vi "Multi_Run_Prog.vi"(0 "Command filename":path, 1 "Setup mode":T9(ring)) -> ()   [LabVIEW 2013]
uses:
  Anemometry Sub Vis/Gen Trav/Traverse_cluster.ctl
  Anemometry Sub Vis/Gen Trav/Spacing.ctl
  Anemometry Sub Vis/Controls/Multi_run_mode.ctl
  Anemometry Sub Vis/Gen Trav/Route mapping/Route_Display_Mode.ctl
  Anemometry Sub Vis/Controls/User_Specific_mode.ctl
  Anemometry Sub Vis/Controls/Multi_Run_Case.ctl
  Anemometry Sub Vis/Gen Trav/Multi_Run_Status.ctl
  Anemometry Sub Vis/Controls/Tunnel_Coordinates.ctl
  Anemometry Sub Vis/Controls/Post_Process.ctl
  ADAM Client/Sub VIs/ADAM Controls/Traverse_Level_State.ctl
  ADAM Client/Sub VIs/ADAM Controls/Tunnel_speed_mode.ctl
  Anemometry Sub Vis/Controls/Overhead.ctl
  ADAM Client/Sub VIs/ADAM Controls/Remember_value_mode.ctl
  Anemometry Sub Vis/Gen Trav/Trav_mode.ctl
  ADAM Client/Sub VIs/ADAM Controls/Client_Source_Status.ctl
  ADAM Client/Sub VIs/ADAM Controls/Update_scan_value.ctl
  Anemometry Sub Vis/File/Setup_Filetype.ctl
  Anemometry Sub Vis/Globals/Meas_global.vi
  Anemometry Sub Vis/Globals/Trav_pos_global.vi
  Anemometry Sub Vis/Globals/Preference_global.vi
  Anemometry Sub Vis/Gen Trav/Route mapping/Route_mapping_global.vi
  ADAM Serial/Instrument drivers/Traverses/~subVIs/DriveConfigGlobal.vi
  Anemometry Sub Vis/Globals/Extra_Commands_Global.vi
panel:
  out "Last Row Run":i32
  in  "Stop after Repeats":bool
  in  "Jump Bad Positions":bool
  in  "Work in Tunnel Coordinates?":T1
  out "Current Overhead Factor":dbl format="%.3f"
  out "Estimated Completion time":string
  out "Max Tunnel Speed":dbl format="%.2f"
  out "Pause message":string
  in  "Pause":bool
  out "Non Starter":bool
  out "No of Rows":i32
  out "Status":T2
  in  "Synchronization Start No":i32=1 min=1 max=100
  out "Multi Run Case":T3
  out "Simulate/Run":T4
  in  "Display Mode":T5=enum."Display View on Crash"
  in  "stop":bool
  out "Currently on Row":i32
  in  "Table":T6[](array[typedef]) {"Row Duration (mins)" format="%#.1f"; "Row No" min=0; "Trace Gas Concentration (%)" min=0.0 format="%#.2f"; "Emission Rate (l/min)" format="%#.2f"; "Tunnel Speed" format="%#.2f"; "Start X" format="%#.2f"; "Start Y" format="%#.2f"; "Start Z" format="%#.2f"; "End X" format="%#.2f"; "End Y" format="%#.2f"; "End Z" format="%#.2f"; "Averaging time (min)" min=0.0 format="%#.2f"}
  # "X           Y            Z"
  # "Start"
  # "End"
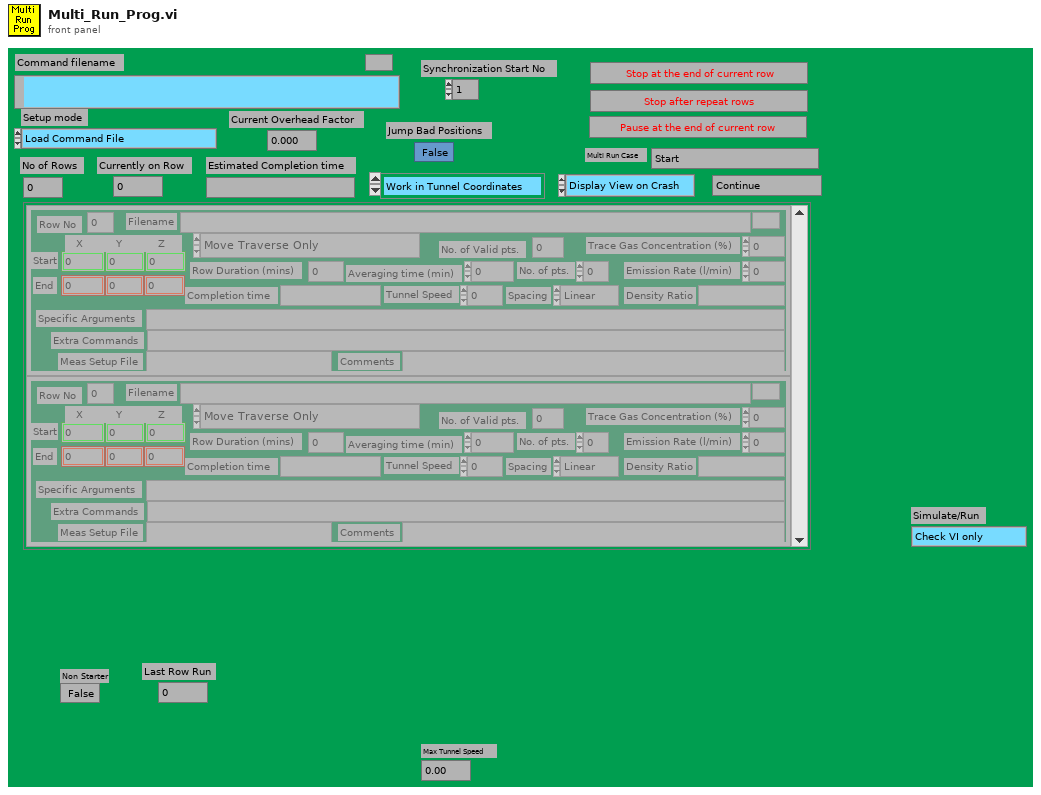
[diagram p1: front panel]
types:
  T1 = typedef "Tunnel_Coordinates.ctl" = enum16{"Work in Tunnel Coordinates", "Work in Model Coordinates"}
  T2 = typedef "Multi_Run_Status.ctl" = enum16{"Continue", "Jump to Next Point", "Jump to Next Row", "Jump To Fall Back", "Terminate Run"}
  T3 = typedef "Multi_Run_Case.ctl" = enum16{"Start", "Load Setup From File", "Has file been edited in Excel?", "Check Max Tunnel Speed", "Pre Check Row", "Check Rows", "Remove blank end rows", "Do results files already exist?", "FFID Bkgnd Measurements?", "First Save Setup file", "Setup Route checking", "Initialise Measurement Prog", "Input Current Position", "Experimental setup control", "Check source flowrates", "Setup for running mode", "Skip Blank Rows", "Which row to execute next", "Evaluate IF Statement", "Perform Measurement Setup", "Set Measurement Conditions", "Execute Row", "Calculate Row TIme", "Update time estimate", "Pause Multi Run Program", "Do Another Row?", "Find Next Fall Back Row", "Shut down source etc", "Email results to users", "Save run efficiency", "Remove Skipped Commands", "Show jumped positions", "Save Setup to File", "End"}
  T4 = typedef "User_Specific_mode.ctl" = enum16{"Check VI only", "Run VI"}
  T5 = typedef "Route_Display_Mode.ctl" = enum16{"Display View Always", "Display View on Crash"}
  T6 = typedef "Traverse_cluster.ctl" = cluster{"Start X":dbl, "Start Y":dbl, "Start Z":dbl, "End X":dbl, "End Y":dbl, "End Z":dbl, "No. of pts.":i32, "Spacing":T7, "Filename":path, "Tunnel Speed":dbl, "Averaging time (min)":dbl, "Extra Commands":string, "Specific Arguments":string, "Emission Rate (l/min)":dbl, "Trace Gas Concentration (%)":dbl, "Density Ratio":string, "Comments":string, "Row No":i32, "Row Type Selector":T8, "Completion time":string, "Row Duration (mins)":dbl, "No. of Valid pts.":i32, "Meas Setup File":string}
  T7 = typedef "Spacing.ctl" = enum16{"Linear", "Log", "Gauss", "Specified", "N/A"}
  T8 = typedef "Multi_run_mode.ctl" = enum16{"Move Traverse Only", "Set Tunnel Speed Only", "Set Source Only", "Set Measurement Conditions", "Single Measurement", "Vertical Profile", "Lateral Profile", "Longitudinal Profile", "Explore Volume", "Multi-Axis Profile", "Auto Calibrate", "Meas Fast FID Bkgnd", "Check Beam Power", "Scanning Valve Measurement", "Run VI Named:", "Set ADAM Ch", "Wait (minutes)", "Send Message", "Synchronize With:", "Fall Back to this Row", "Turn Off Row Repeating", "Blank Row", "Traverse 3D Volume"}
  T9 = enum16{"Load Command File", "Save Command File", "Check Multi Run Prog", "Check Multi Run Prog With Live Moves", "Run Multi Run Prog"}
  T10 = typedef "Post_Process.ctl" = enum16{"Take New Data", "Post Process Raw Data File"}
  T11 = typedef "Traverse_Level_State.ctl" = enum16{"Running", "Complete"}
  T12 = enum32{"existing file", "new file", "new or existing file", "existing dir", "new dir", "new or existing dir", "existing file (use LLBs)", "new file (use LLBs)", "new or existing file (use LLBs)", "new or existing file or directory (use LLBs)"}
  T13 = typedef "Tunnel_speed_mode.ctl" = enum16{"Set Speed", "Set Speed then wait", "Is tunnel speed allowable?"}
  T14 = enum16{"All Channel Names", "Valid Channel Names"}
  T15 = typedef "Overhead.ctl" = enum16{"Update total times", "Read Current Overhead", "Re Scale totals to 3 hrs", "Initialise totals to 3hr"}
  T16 = typedef "Remember_value_mode.ctl" = enum16{"Read only", "Read and Write"}
  T17 = typedef "Trav_mode.ctl" = enum16{"Move traverse", "Read traverse position", "Teach Position"}
  T18 = typedef "Client_Source_Status.ctl" = enum16{"Not Using", "Using", "Must Have"}
  T19 = typedef "Update_scan_value.ctl" = cluster{"Channel Name":string, "New Value":dbl}
  T20 = typedef "Setup_Filetype.ctl" = enum16{"Measurement Setups", "Calibration Setups", "General", "Results File Plotter Setups", "Speed Calib Tweaks"}
  T21 = typedef "AxisConfigCluster.ctl" = cluster{"Channel Properties":T22, "Static Drive Configuration":T23}
  T22 = typedef "DriveProperties.ctl" = cluster{"Channel Name":string, "Vel. Default":dbl, "Acc. Default":dbl, "Vel. Max":dbl, "Vel. Min":dbl, "Acc. Max":dbl, "Acc. Min":dbl, "Pulses/unit":dbl, "Address":u8, "Pulse Offset":i32, "Pos Tolerance":dbl, "Pulses/rev":dbl, "Backlash/Eng units":dbl, "Current Pos":dbl, "Ch Status":enum16{"Active", "Offline", "Simulate"}, "Port Name":string, "Axis Transform mode":string, "Metadata Ch Name":string, "Type":string}
  T23 = typedef "DriveStaticConfig.ctl" = cluster{"Correction Gain % (CG)":u16, "Dead Band (DB)":i32, "Dead Band Window (DW)":i32, "Encoder Resolution (ER)":i32, "Step Mode  (FSB)":u16, "Position Maintenance (FSC)":u16, "Stop on Stall (FSD)":u16, "Activate OP1 on stall (FSE)":u16, "Stop on Trigger 3 (FSF)":u16, "OP2 in Deadband (FSG)":u16, "Stall Detect (FSH)":u16, "Limit Disable (LD)":u16, "Motor Resolution (MR)":enum16{"200", "400", "1000", "2000", "4000", "5000", "10000", "12800", "18000", "20000", "21600", "25000", "25400", "25600", "36000", "50000", "278528", "425984", "507904", "614400", "655360", "819200", "1024000"}, "Limit Switch Sense (OSA)":u16, "Home Position (OSB)":u16, "Home Switch Sense (OSC)":u16, "Encoder Z for Home (OSD)":u16, "Reference edge of Home (OSH)":u16, "RS232 Echo Control (SSA)":u16, "Buffer at Limit (SSG)":u16, "Buffer at Stop (SSH)":u16, "Indexer Mode  (FSA)":u16, "Type":string, "ConfigString":string, "De Power Motor":enum16{"TRUE", "FALSE"}}
  T24 = typedef "Status_Cluster.ctl" = cluster{"Status":T2, "Error Type":string, "Error Description":string}
  T25 = typedef "Server_Comms.ctl" = enum16{"Server Link Healthy", "Do Not Link To Server"}
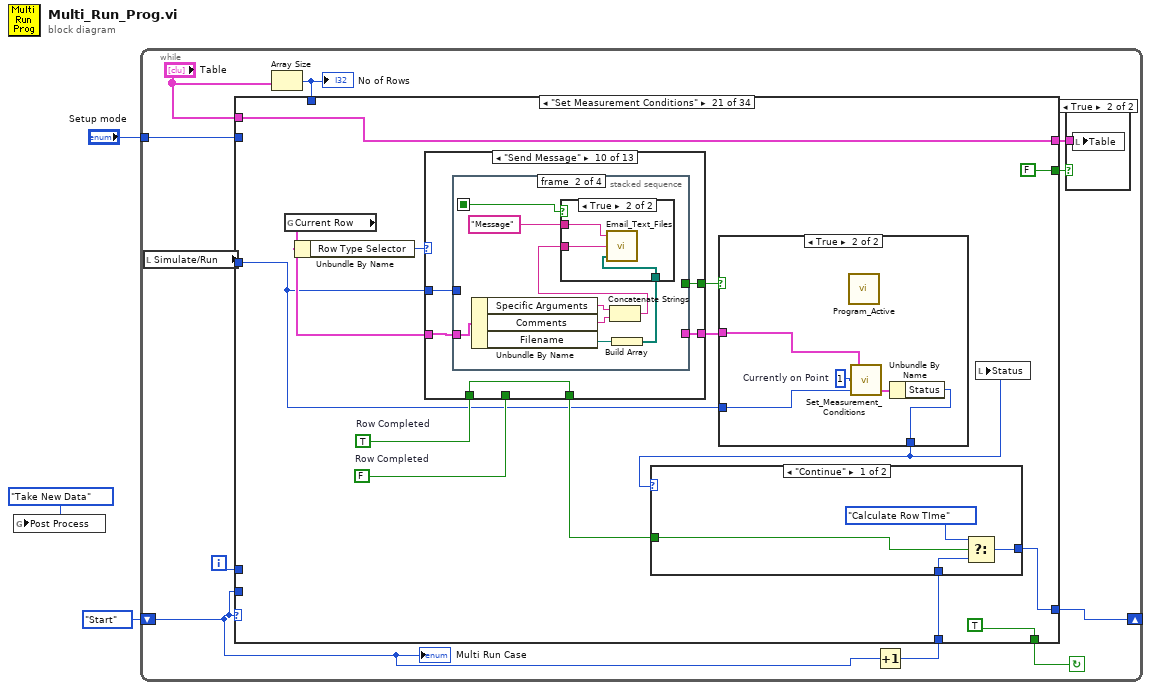
[diagram p0: block diagram]
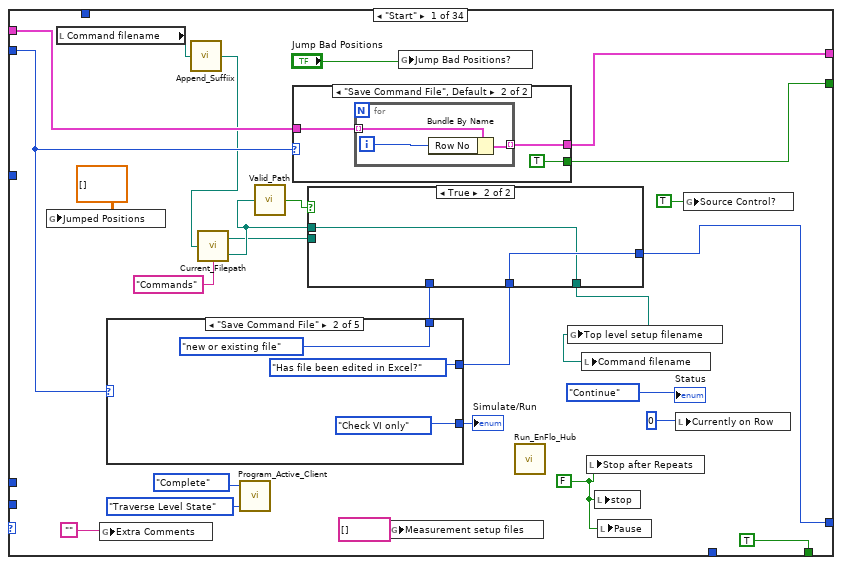
[diagram p3: hidden frame]
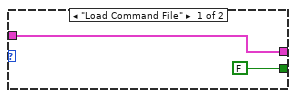
[diagram p4: hidden frame]
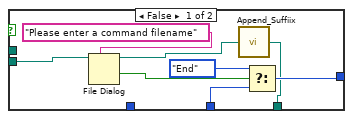
[diagram p5: hidden frame]
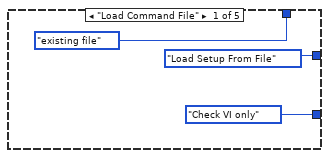
[diagram p6: hidden frame]
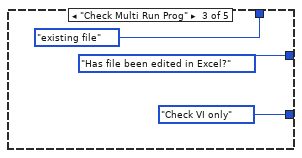
[diagram p7: hidden frame]
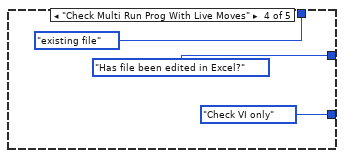
[diagram p8: hidden frame]
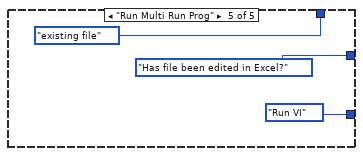
[diagram p9: hidden frame]
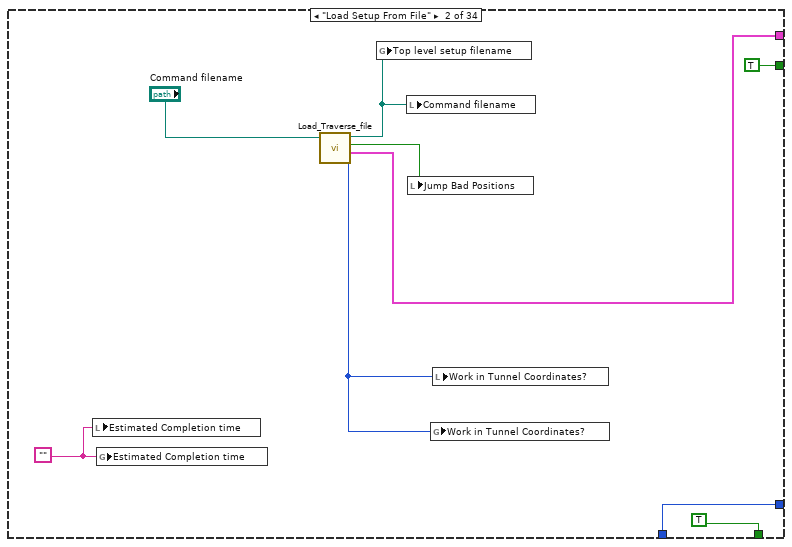
[diagram p10: hidden frame]
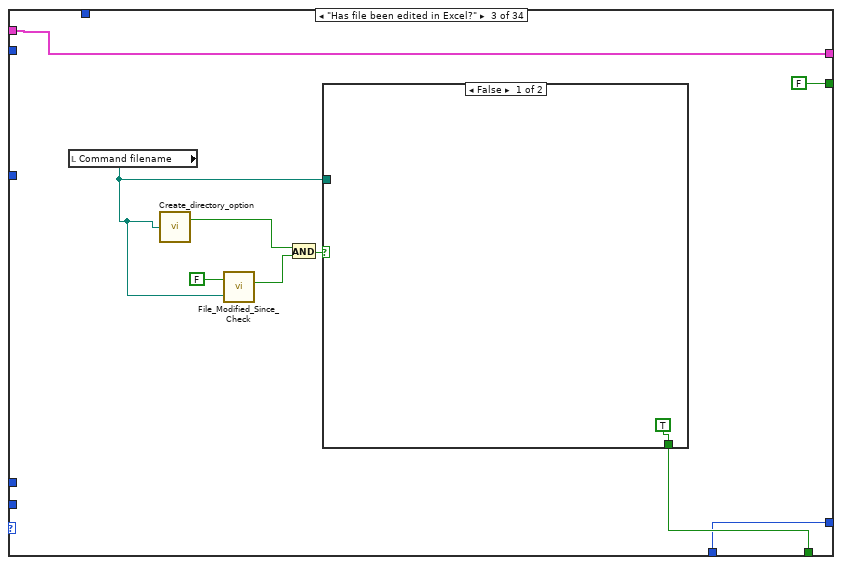
[diagram p11: hidden frame]
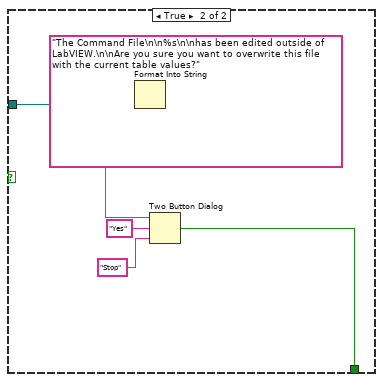
[diagram p12: hidden frame]
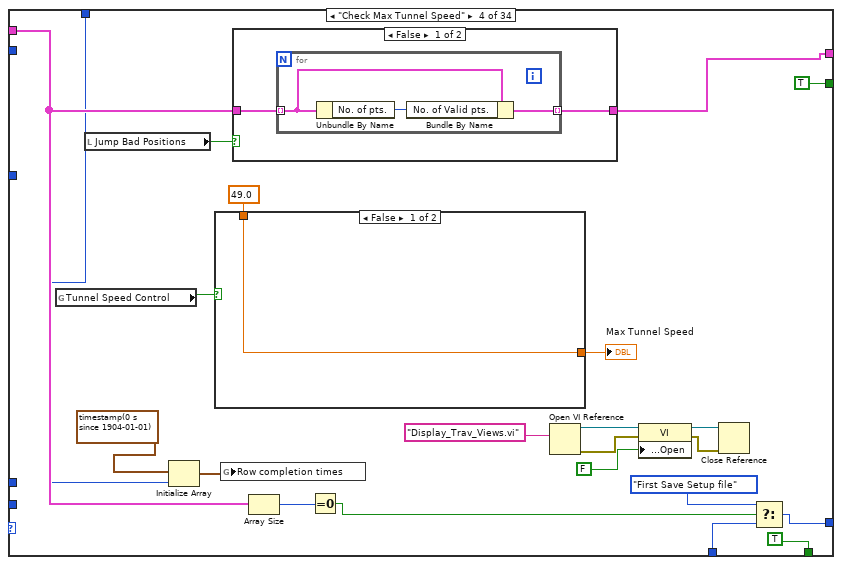
[diagram p13: hidden frame]
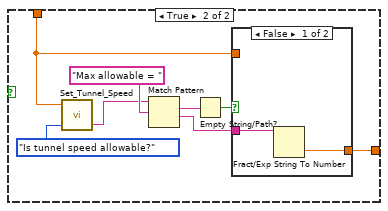
[diagram p15: hidden frame]
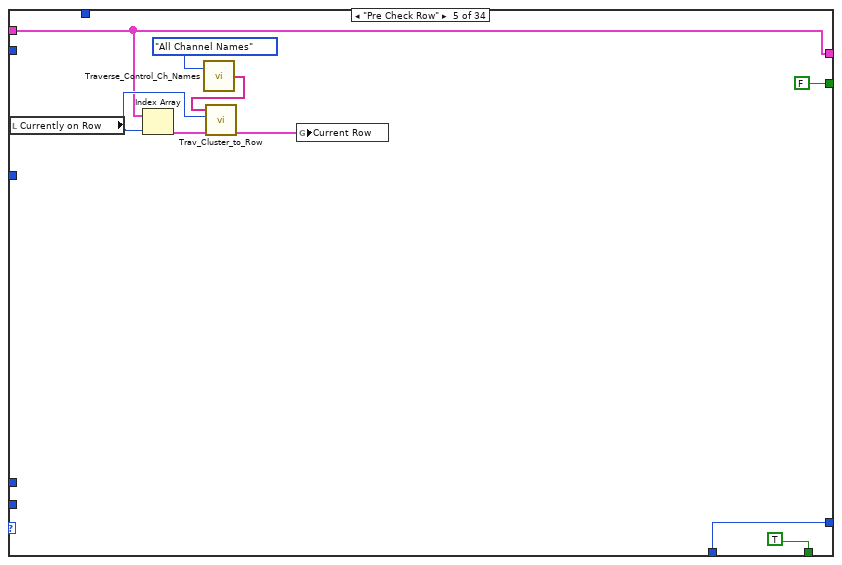
[diagram p17: hidden frame]
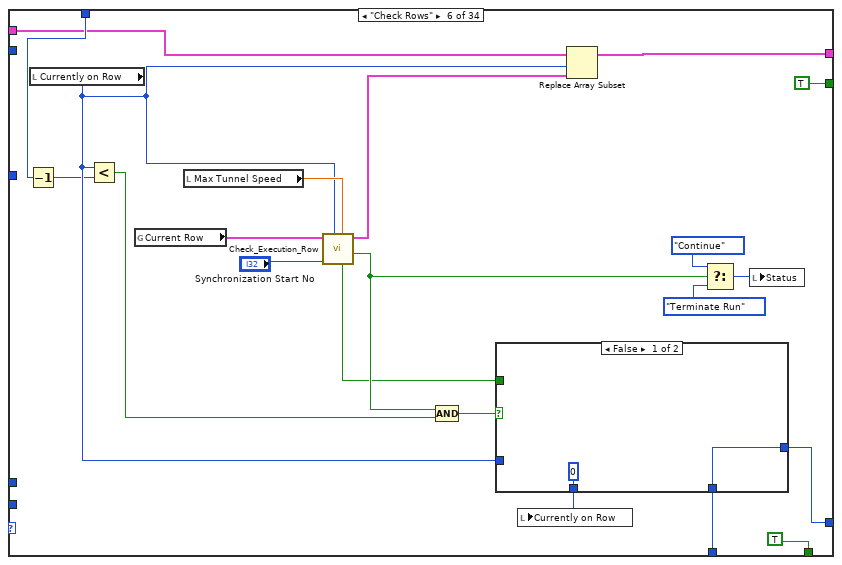
[diagram p18: hidden frame]
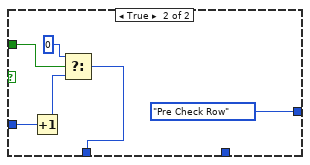
[diagram p19: hidden frame]
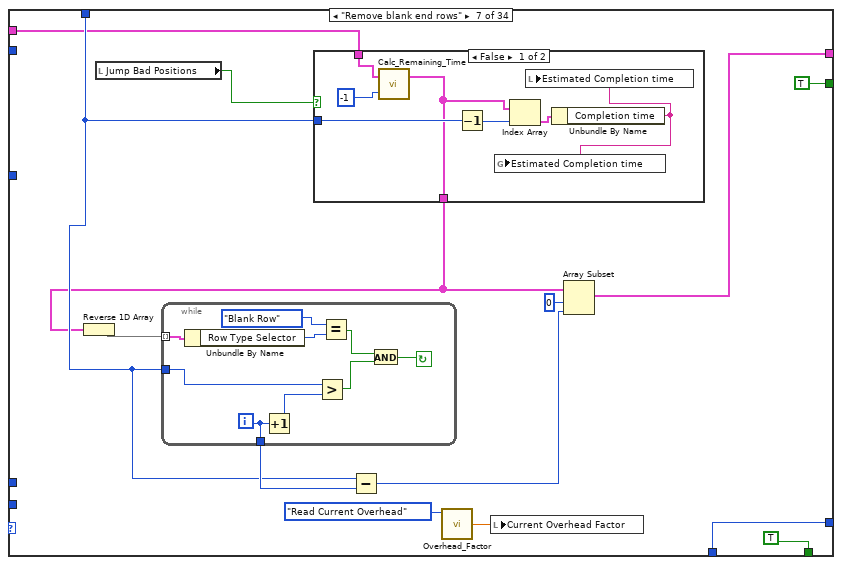
[diagram p20: hidden frame]
diagram:
  n1 = global write "Meas_global.vi" "Post Process"(Post_Process."Take New Data" ("Post Process")) -> ()
  n2 = while {
    shift-left: Multi_Run_Case."Start" ("Multi Run Case") -> [w10]
    shift-right: [w6] -> _
    tunnel: "Setup mode" -> [w13]
    i -> [w11]
    stop <- w14 continue-if-true
    n3 = local read "Simulate/Run"() -> (w7:T4)
    n4 = Array Size(array="Table") -> (size(s)=w5:i32)
    "No of Rows" <- w5
    n5 = Increment(x=w10) -> (x+1=w12:T3)
    n6 = case shown="\"Set Measurement Conditions\"" w10 {
      tunnel: [TRUE TRUE w87 TRUE TRUE TRUE TRUE TRUE TRUE TRUE TRUE ("Continue?") TRUE ("Continue?") TRUE TRUE TRUE w506 TRUE ("Continue?") TRUE ("Continue?") TRUE TRUE ("Continue?") TRUE TRUE TRUE TRUE TRUE TRUE TRUE TRUE TRUE TRUE TRUE TRUE TRUE FALSE] -> w14
      tunnel: w13 -> [w26 _ _ _ _ _ _ _ _ w395 _ _ _ _ _ _ _ _ _ _ _ _ _ _ _ _ _ _ _ _ _ _ w1254 _]
      tunnel: "Table" -> [w39 _ w84 w114 w142 w154 w179 w210 w368 w397 w419 w472 w477 w483 w493 w509 w580 w624 w740 w791 w803 w896 w932 w964 w1007 w1053 w1101 w1131 w1152 w1199 w1204 w1213 w1275 w1339]
      tunnel: w7 -> [_ _ _ _ _ _ _ w209 _ _ _ _ _ w487 w492 w508 _ w622 w737 w788 w801 w895 w930 w961 _ w1062 _ w1122 _ _ _ _ w1265 _]
      tunnel: w10 -> [_ _ _ _ _ _ _ _ _ _ _ _ _ _ _ _ _ _ _ _ _ _ _ _ _ _ _ _ _ _ _ _ _ _]
      tunnel: w12 -> [_ w80 w86 w112 w146 w156 w190 w214 w363 w394 w423 w470 w478 w482 w498 w511 w582 w620 w745 w792 w810 w893 w922 w966 w1010 _ _ w1115 w1154 w1201 w1207 w1221 w1273 w1338]
      tunnel: w11 -> [_ _ _ _ _ _ _ _ _ _ _ _ _ _ _ _ _ _ _ _ _ _ _ _ w1008 _ _ _ _ _ _ _ _ _]
      tunnel: [w37 w80 w86 w111 w146 w155 w190 w214 w363 w390 w423 w469 w478 w482 w495 w511 w582 w621 w744 w792 w811 w893 w922 w966 w1011 w1045 w1098 w1126 w1154 w1201 w1207 w1221 w1273 w1338] -> w6
      tunnel: [w25 TRUE FALSE ("Rows Added ?") TRUE ("Rows Added ?") FALSE TRUE TRUE FALSE FALSE TRUE FALSE FALSE FALSE FALSE FALSE TRUE FALSE ("Rows Added ?") FALSE ("Rows Added ?") FALSE FALSE ("Rows Added ?") FALSE FALSE FALSE TRUE ("Rows Added ?") FALSE FALSE FALSE FALSE FALSE FALSE TRUE TRUE TRUE FALSE] -> w8
      tunnel: w5 -> [_ _ _ w106 _ w160 w181 _ _ _ _ _ _ _ _ _ w583 w623 _ _ _ _ _ w960 _ w1048 _ _ _ _ _ _ _ _]
      tunnel: [w38 w81 w84 w116 w142 w163 w185 w210 w368 w398 w419 w472 w477 w483 w493 w507 w580 w625 w740 w791 w803 w896 w932 w963 w1007 w1053 w1101 w1131 w1152 w1199 w1203 w1213 w1274 w1339] -> w4
      frame "Start" {
        w23 = FALSE ("Measurment setup Found?")
        n7 = global write "Trav_pos_global.vi" "Jumped Positions"(dbl[][] [] ("Jumped Positions")) -> ()
        n8 = local read "Command filename"() -> (w29:path)
        n9 = global write "Meas_global.vi" "Extra Comments"("") -> ()
        n10 = case shown="\"Save Command File\"" w26 {
          tunnel: [User_Specific_mode."Check VI only" ("Simulate/Run") User_Specific_mode."Check VI only" ("Simulate/Run") User_Specific_mode."Check VI only" ("Simulate/Run") User_Specific_mode."Check VI only" ("Simulate/Run") User_Specific_mode."Run VI" ("Simulate/Run")] -> w40
          tunnel: [Multi_Run_Case."Load Setup From File" ("Multi Run Case") Multi_Run_Case."Has file been edited in Excel?" ("Multi Run Case") Multi_Run_Case."Has file been edited in Excel?" ("Multi Run Case") Multi_Run_Case."Has file been edited in Excel?" ("Multi Run Case") Multi_Run_Case."Has file been edited in Excel?" ("Multi Run Case")] -> w36
          tunnel: [T12."existing file" ("select mode (2)") T12."new or existing file" ("select mode (2)") T12."existing file" ("select mode (2)") T12."existing file" ("select mode (2)") T12."existing file" ("select mode (2)")] -> w24
          frame "Load Command File" {
          }
          frame "Save Command File" {
          }
          frame "Check Multi Run Prog" {
          }
          frame "Check Multi Run Prog With Live Moves" {
          }
          frame "Run Multi Run Prog" {
          }
        }
        "Simulate/Run" <- w40
        n11 = call "Append_Suffiix.vi"("Results file"=w29) -> ("appended path"=w18:path)
        n12 = call "Current_Filepath.vi"("Filename in"=w18, "Data Type"="Commands") -> ("Filename Out"=w17:path, "Directory"=w16:path)
        n13 = call "Program_Active_Client.vi"("Mode"=enum16{"Program Active", "Traverse Level State"}."Traverse Level State", "Traverse level State"=Traverse_Level_State."Complete") -> ()  [unwired: 1 in, 3 out]
        n14 = call "Valid_Path.vi"("Filename"=w17) -> ("Valid Path?"=w27:bool)
        n15 = case shown="\"Save Command File\", Default" w26 {
          tunnel: w39 -> [w43 w46]
          tunnel: [w43 w45] -> w38
          tunnel: [FALSE TRUE] -> w25
          frame "Load Command File" {
          }
          frame "Save Command File", Default {
            n16 = for {
              tunnel: w46 -> [w49] mode=indexing
              tunnel: [w48] -> w45 mode=indexing
              i -> [w47]
              n17 = Bundle By Name(cluster=w49, "Row No"=w47) -> (w48:T6)
            }
          }
        }
        n18 = case shown="True" w27 {
          tunnel: [w55 w59] -> w37
          tunnel: w36 -> [w56 w59]
          tunnel: w17 -> [_ w58]
          tunnel: [w54 w58] -> w28
          tunnel: w24 -> [_ _]
          tunnel: w16 -> [w50 _]
          frame False {
            n19 = File Dialog(7:"Please enter a command filename" ("prompt"), 11:w50) -> (1:w52:bool, 3:w53:path)  [unwired: 1 in, 6 out]
            n20 = call "Append_Suffiix.vi"("Results file"=w53) -> ("appended path"=w54:path)
            n21 = Select(t=Multi_Run_Case."End" ("Multi Run Case"), s=w52, f=w56) -> (s? t:f=w55:T3)
          }
          frame True {
          }
        }
        n22 = global write "Trav_pos_global.vi" "Measurement setup files"(string[] [] ("Measurement setup files")) -> ()
        n23 = global write "Trav_pos_global.vi" "Jump Bad Positions?"("Jump Bad Positions") -> ()
        n24 = call "Run_EnFlo_Hub.vi"() -> ()  [unwired: 8 out]
        n25 = global write "Trav_pos_global.vi" "Top level setup filename"(w28) -> ()
        n26 = local write "Command filename"(w28) -> ()
        n27 = local write "Stop after Repeats"(w23) -> ()
        n28 = local write "stop"(w23) -> ()
        n29 = local write "Pause"(w23) -> ()
        n30 = local write "Currently on Row"(0 ("Currently on Row")) -> ()
        n31 = global write "Trav_pos_global.vi" "Source Control?"(TRUE ("Source Control?")) -> ()
        "Status" <- Multi_Run_Status."Continue" ("Status")
      }
      frame "Load Setup From File" {
        w76 = ""
        n32 = local write "Estimated Completion time"(w76) -> ()
        n33 = global write "Trav_pos_global.vi" "Estimated Completion time"(w76) -> ()
        n34 = call "Load_Traverse_file.vi"("Setup filename"="Command filename") -> ("Setup filename Out"=w78:path, "Jump Bad Positions"=w75:bool, "Table"=w81:T6[], "Work in Tunnel Coordinates?"=w77:T1)  [unwired: 2 out]
        n35 = global write "Trav_pos_global.vi" "Top level setup filename"(w78) -> ()
        n36 = local write "Command filename"(w78) -> ()
        n37 = local write "Jump Bad Positions"(w75) -> ()
        n38 = global write "Trav_pos_global.vi" "Work in Tunnel Coordinates?"(w77) -> ()
        n39 = local write "Work in Tunnel Coordinates?"(w77) -> ()
      }
      frame "Has file been edited in Excel?" {
        n40 = local read "Command filename"() -> (w88:path)
        n41 = call "Create_directory_option.vi"("Filename"=w88) -> ("Path is to existing File"=w91:bool)  [unwired: 1 out]
        n42 = call "File_Modified_Since_Check.vi"("Pathname"=w88, "Just Modified?"=FALSE) -> ("Modified?"=w90:bool)
        n43 = And(x=w91, y=w90) -> (x .and. y?=w92:bool)
        n44 = case shown="False" w92 {
          tunnel: w88 -> [_ w99]
          tunnel: [TRUE ("T button?") w94] -> w87
          frame False {
          }
          frame True {
            n45 = Format Into String(format string="The Command File\n\n%s\n\nhas been edited outside of LabVIEW.\n\nAre you sure you want to overwrite this file  with the current table values?" ("Format String"), w99) -> (resulting string=w97:string)  [unwired: 2 in, 1 out]
            n46 = Two Button Dialog(message=w97, 1:"Stop" ("F button name (\"Cancel\")"), 2:"Yes" ("T button name (\"OK\")")) -> (T button?=w94:bool)
          }
        }
      }
      frame "Check Max Tunnel Speed" {
        n47 = global read "Preference_global.vi" "Tunnel Speed Control"() -> (w117:bool)
        n48 = local read "Jump Bad Positions"() -> (w115:bool)
        n49 = Initialize Array(timestamp(0 s since 1904-01-01) ("seconds since 1Jan1904"), w106) -> (w107:timestamp[])
        n50 = case shown="False" w117 {
          tunnel: 49.0 ("Tunnel Velocity m/s") -> [w128 w129]
          tunnel: [w128 w131] -> w119
          frame False {
          }
          frame True {
            n51 = call "Set_Tunnel_Speed.vi"("Mode"=Tunnel_speed_mode."Is tunnel speed allowable?", "Tunnel Velocity m/s"=w129) -> ("Error String"=w134:string)  [unwired: 1 in, 2 out]
            n52 = Match Pattern(string=w134, regular expression="Max allowable = ") -> (match substring=w133:string, after substring=w130:string)  [unwired: 3 out]
            n53 = Empty String/Path?(string/path=w133) -> (empty?=w132:bool)
            n54 = case shown="False" w132 {
              tunnel: [w137 w139] -> w131
              tunnel: w129 -> [_ w139]
              tunnel: w130 -> [w138 _]
              frame False {
                n55 = Fract/Exp String To Number(string=w138) -> (number=w137:dbl)  [unwired: 4 out]
              }
              frame True {
              }
            }
          }
        }
        "Max Tunnel Speed" <- w119
        n56 = global write "Trav_pos_global.vi" "Row completion times"(w107) -> ()
        n57 = case shown="False" w115 {
          tunnel: w114 -> [w123 w127]
          tunnel: [w122 w127] -> w116
          frame False {
            n58 = for {
              tunnel: w123 -> [w125] mode=indexing
              tunnel: [w124] -> w122 mode=indexing
              n59 = Unbundle By Name(w125) -> ("No. of pts."=w126:i32)
              n60 = Bundle By Name(cluster=w125, "No. of Valid pts."=w126) -> (w124:T6)
            }
          }
          frame True {
          }
        }
        n61 = Array Size(array=w114) -> (size(s)=w113:i32)
        n62 = Equal To 0?(x=w113) -> (x = 0?=w110:bool)
        n63 = Open VI Reference(vi path="Display_Trav_Views.vi" ("VI path")) -> (vi reference=w105:refnum<vi>, error out=w104:errorcluster)  [unwired: 1 in, 4 out]
        n64 = property class="VI"(reference=w105, error in=w104, "Front Panel Window:Open"=FALSE) -> (reference out=w102:refnum<vi>, error out=w101:errorcluster)
        n65 = Close Reference(reference=w102, error in (no error)=w101) -> ()  [unwired: 1 out]
        n66 = Select(t=Multi_Run_Case."First Save Setup file" ("Multi Run Case"), s=w110, f=w112) -> (s? t:f=w111:T3)
      }
      frame "Pre Check Row" {
        n67 = local read "Currently on Row"() -> (w143:i32)
        n68 = Index Array(array=w142, index=w143) -> (element=w144:T6)
        n69 = call "Traverse_Control_Ch_Names.vi"("Mode"=T14."All Channel Names") -> ("Channel names"=w140:string[])  [unwired: 1 in]
        n70 = call "Trav_Cluster_to_Row.vi"("Traverse line in"=w144, "Row Number"=w143, "Channel names"=w140) -> ("Traverse line Out"=w145:T6)  [unwired: 4 out]
        n71 = global write "Trav_pos_global.vi" "Current Row"(w145) -> ()
      }
      frame "Check Rows" {
        n72 = Decrement(x=w160) -> (x-1=w151:i32)
        n73 = local read "Currently on Row"() -> (w152:i32)
        n74 = Less?(x=w152, y=w151) -> (x < y?=w159:bool)
        n75 = global read "Trav_pos_global.vi" "Current Row"() -> (w149:T6)
        n76 = local read "Max Tunnel Speed"() -> (w162:dbl)
        n77 = call "Check_Execution_Row.vi"("Execution Row"=w149, "Synchronization Start No"="Synchronization Start No", "Row Index"=w152, "Max Tunnel Speed"=w162) -> ("Editted Row"=w150:bool, "Execution Row Out"=w153:T6, "Continue?"=w161:bool)  [unwired: 1 in, 3 out]
        n78 = Compound Arithmetic op=AND(w161, w159) -> (w158:bool)
        n79 = case shown="False" w158 {
          tunnel: [0 w173] -> w157
          tunnel: w152 -> [_ w177]
          tunnel: w156 -> [w171 _]
          tunnel: [w171 Multi_Run_Case."Pre Check Row" ("Multi Run Case")] -> w155
          tunnel: w150 -> [_ w175]
          frame False {
          }
          frame True {
            n80 = Increment(x=w177) -> (x+1=w174:i32)
            n81 = Select(t=0, s=w175, f=w174) -> (s? t:f=w173:i32)
          }
        }
        n82 = local write "Currently on Row"(w157) -> ()
        n83 = Replace Array Subset(array=w154, new element=w153, index=w152) -> (w163:T6[])
        n84 = Select(t=Multi_Run_Status."Continue" ("Status"), s=w161, f=Multi_Run_Status."Terminate Run" ("Status")) -> (s? t:f=w167:T2)
        n85 = local write "Status"(w167) -> ()
      }
      frame "Remove blank end rows" {
        n86 = local read "Jump Bad Positions"() -> (w178:bool)
        n87 = case shown="False" w178 {
          tunnel: w181 -> [w196 _]
          tunnel: w179 -> [w195 w199]
          tunnel: [w193 w199] -> w180
          frame False {
            n88 = call "Calc_Remaining_Time.vi"("Currently on Row"=-1 ("Start Index"), "Table In"=w195) -> ("Table Out"=w193:T6[])  [unwired: 1 out]
            n89 = Decrement(x=w196) -> (x-1=w198:i32)
            n90 = Index Array(array=w193, index=w198) -> (element=w197:T6)
            n91 = Unbundle By Name(w197) -> ("Completion time"=w192:string)
            n92 = global write "Trav_pos_global.vi" "Estimated Completion time"(w192) -> ()
            n93 = local write "Estimated Completion time"(w192) -> ()
          }
          frame True {
          }
        }
        n94 = Reverse 1D Array(array=w180) -> (reversed array=w189:T6[])
        n95 = while {
          tunnel: [w200] -> w187
          tunnel: w181 -> [w204]
          tunnel: w189 -> [w208] mode=indexing
          i -> [w200]
          stop <- w201 continue-if-true
          n96 = Unbundle By Name(w208) -> ("Row Type Selector"=w206:T8)
          n97 = Increment(x=w200) -> (x+1=w205:i32)
          n98 = Greater?(x=w204, y=w205) -> (0:w203:bool)
          n99 = Equal?(x=Multi_run_mode."Blank Row" ("Row Type Selector"), y=w206) -> (x = y?=w202:bool)
          n100 = And(x=w202, y=w203) -> (x .and. y?=w201:bool)
        }
        n101 = Subtract(x=w181, y=w187) -> (x-y=w186:i32)
        n102 = call "Overhead_Factor.vi"("Mode"=Overhead."Read Current Overhead") -> ("Current Overhead Factor"=w182:dbl)  [unwired: 3 in]
        n103 = local write "Current Overhead Factor"(w182) -> ()
        n104 = Array Subset(array=w180, index=0 ("Array Index"), length=w186) -> (w185:T6[])
      }
      frame "Do results files already exist?" {
        n105 = for {
          tunnel: w210 -> [w226] mode=indexing
          tunnel: [w224] -> w216 mode=indexing
          shift-right: [w220] -> _
          shift-left: path[] [] -> [w221]
          tunnel: w209 -> [w218]
          n106 = Unbundle By Name(w226) -> ("Specific Arguments"=w217:string, "Emission Rate (l/min)"=w225:dbl, "Row Type Selector"=w223:T8, "Filename"=w222:path)
          n107 = while {
            shift-left: w221 -> [w234]
            shift-right: [w233] -> w220
            tunnel: w222 -> [w235]
            tunnel: w223 -> [w239]
            shift-left: 0 -> [w240]
            shift-right: [w236] -> _
            tunnel: w218 -> [w230]
            shift-right: [w229] -> _
            shift-left: _ -> [w228]
            tunnel: w217 -> [w227]
            stop <- w238 continue-if-true
            n108 = Increment(x=w240) -> (x+1=w237:i32)
            n109 = case shown="0, Default" w240 {
              tunnel: w239 -> [w249 _ _ _ _ _ _ _ _ _ _ _]
              tunnel: [w244 w269 w274 w281 w286 TRUE ("exists?") TRUE ("exists?") FALSE ("exists?") FALSE ("exists?") TRUE ("true") w343 w356] -> w238
              tunnel: w237 -> [w251 w272 w277 w280 w287 w292 w303 w314 w325 w329 w341 _]
              tunnel: [w251 w272 w277 w280 w287 w290 w302 w314 w325 w330 w341 w355] -> w236
              tunnel: [w250 w271 w276 w279 w284 w300 w311 w316 w318 w327 w345 w361] -> w233
              tunnel: w234 -> [w250 w271 w276 w279 w285 w300 w311 w316 w318 w327 w345 w361]
              tunnel: w235 -> [w243 _ _ _ _ _ _ _ _ _ _ _]
              tunnel: 7 -> [_ _ _ _ _ _ _ _ _ w328 _ w355]
              tunnel: 9 -> [_ _ _ _ _ w291 _ _ _ _ _ _]
              tunnel: w230 -> [_ _ _ _ _ _ _ _ _ _ w344 _]
              tunnel: [w242 w268 w273 w278 w283 w288 w301 w312 w317 w326 w342 w354] -> w229
              tunnel: w228 -> [_ w268 w273 w278 w283 w288 w301 w312 w317 w326 w342 w354]
              tunnel: w227 -> [w241 _ _ _ _ _ _ _ _ _ _ _]
              frame 0, Default {
                n110 = case shown="\"Send Message\"" w249 {
                  tunnel: [TRUE w259 FALSE FALSE] -> w246
                  tunnel: w243 -> [w252 w258 w264 w266]
                  tunnel: w241 -> [_ w256 _ _]
                  tunnel: [w252 w258 w264 w266] -> w242
                  frame "Move Traverse Only", Default {
                  }
                  frame "Run VI Named:" {
                    n111 = Match Pattern(string=w256, regular expression=";") -> (before substring=w255:string)  [unwired: 4 out]
                    n112 = call <vilib>:"Trim Whitespace.vi"("string"=w255) -> ("trimmed string"=w254:string)  [unwired: 1 in]
                    n113 = Equal?(x=w254, y="Pressure_Tapped_Cube.vi") -> (x = y?=w260:bool)
                    n114 = Equal?(x=w254, y="Take_Data_on_the_Move.vi") -> (x = y?=w261:bool)
                    n115 = Or(x=w260, y=w261) -> (x .or. y?=w259:bool)
                  }
                  frame "Auto Calibrate" {
                  }
                  frame "Send Message" {
                  }
                }
                n116 = local read "Status"() -> (w247:T2)
                n117 = Not Equal?(x=Multi_Run_Status."Terminate Run" ("Status"), y=w247) -> (x != y?=w245:bool)
                n118 = And(x=w246, y=w245) -> (x .and. y?=w244:bool)
              }
              frame 1 {
                n119 = Not Equal?(x=path "", y=w268) -> (x != y?=w269:bool)
              }
              frame 2 {
                n120 = Not Equal?(x=w273, y=path "") -> (x != y?=w274:bool)
              }
              frame 3 {
                n121 = Search 1D Array(1D array=w279, element=w278) -> (index of element=w282:i32)  [unwired: 1 out]
                n122 = Less Than 0?(x=w282) -> (x < 0?=w281:bool)
              }
              frame 4 {
                n123 = Build Array (concatenate)(w285, w283) -> (w284:path[])
                n124 = call "Does_file_exist_(simple).vi"("Pathname"=w283) -> ("exists?"=w286:bool)
              }
              frame 5 {
                n125 = Path To String(path=w288) -> (string=w299:string)
                n126 = global read "Meas_global.vi" "Start Time of experiment"() -> (w294:dbl)
                n127 = Concatenate Strings(w299, "Append" ("Substring")) -> (w297:string)
                n128 = call "Remember_value.vi"("Mode"=Remember_value_mode."Read only", "Ch name"=w297) -> ("Output Value"=w295:dbl)  [unwired: 1 in]
                n129 = Not Equal?(x=w294, y=w295) -> (x != y?=w293:bool)
                n130 = Select(t=w292, s=w293, f=w291) -> (s? t:f=w290:i32)
              }
              frame 6 {
                n131 = Increment(x=w303) -> (x+1=w304:i32)
                n132 = Format Into String(format string="The results filename \"%s\" already exists.\nDo you wish to append to this file during the run?" ("Format String"), w301) -> (resulting string=w308:string)  [unwired: 2 in, 1 out]
                n133 = Two Button Dialog(message=w308, 1:"Abort Run" ("F button name (\"Cancel\")"), 2:"Append" ("T button name (\"OK\")")) -> (T button?=w305:bool)
                n134 = Select(t=w304, s=w305, f=w303) -> (s? t:f=w302:i32)
              }
              frame 7 {
                n135 = local write "Status"(Multi_Run_Status."Terminate Run" ("Status")) -> ()
              }
              frame 8 {
                n136 = Path To String(path=w317) -> (string=w324:string)
                n137 = Concatenate Strings(w324, "Append" ("Substring")) -> (w322:string)
                n138 = global read "Meas_global.vi" "Start Time of experiment"() -> (w319:dbl)
                n139 = call "Remember_value.vi"("Mode"=Remember_value_mode."Read and Write", "Input Value"=w319, "Ch name"=w322) -> ()  [unwired: 1 out]
              }
              frame 9 {
                n140 = call "Read_File_Simple.vi"("Filename"=w326) -> ("string"=w333:string)  [unwired: 2 in, 7 out]
                n141 = call "Is_it_a_Results_File.vi"("character string"=w333) -> ("Results File?"=w332:bool)  [unwired: 2 out]
                n142 = case shown="True" w332 {
                  tunnel: w326 -> [w336 _]
                  tunnel: [w334 w340] -> w330
                  tunnel: w329 -> [_ w340]
                  tunnel: w328 -> [w334 _]
                  frame False {
                    n143 = Path To String(path=w336) -> (string=w338:string)
                    n144 = Format Into String(format string="The File %s is not in the correct Results file format.\nCheck that it is tab delimited rather than excel format, or choose another file." ("Format String"), w338) -> (resulting string=w335:string)  [unwired: 2 in, 1 out]
                    n145 = One Button Dialog(message=w335, button name ("OK")="Stop") -> ()  [unwired: 1 out]
                  }
                  frame True {
                  }
                }
              }
              frame 10 {
                n146 = case shown="\"Check VI only\", Default" w344 {
                  tunnel: w342 -> [_ w353]
                  tunnel: [FALSE ("exists?") w347] -> w343
                  frame "Check VI only", Default {
                  }
                  frame "Run VI" {
                    n147 = call "Open_File_for_write.vi"("append to file? (new file:F)"=TRUE, "file path"=w353) -> ("error out"=w351:errorcluster, "refnum"=w352:refnum<file>)  [unwired: 1 in, 7 out]
                    n148 = Unbundle By Name(w351) -> ("code"=w350:i32)
                    n149 = Close File(refnum=w352, error in=w351) -> ()  [unwired: 2 out]
                    n150 = Equal?(x=10 ("code"), y=w350) -> (x = y?=w347:bool)
                  }
                }
              }
              frame 11 {
                n151 = Path To String(path=w354) -> (string=w359:string)
                n152 = Format Into String(format string="The File %s is already open in another application." ("Format String"), w359) -> (resulting string=w358:string)  [unwired: 2 in, 1 out]
                n153 = One Button Dialog(message=w358, button name ("OK")="Stop") -> (true=w356:bool)
              }
            }
          }
          n154 = Greater Than 0?(x=w225) -> (x > 0?=w224:bool)
        }
        n155 = Or Array Elements(Boolean array=w216) -> (logical OR=w212:bool)
        n156 = global write "Trav_pos_global.vi" "Source Control?"(w212) -> ()
      }
      frame "FFID Bkgnd Measurements?" {
        n157 = for {
          tunnel: w368 -> [w384] mode=indexing
          tunnel: [w372] -> w367 mode=indexing
          tunnel: [w373] -> w366 mode=indexing
          n158 = Unbundle By Name(w384) -> ("Row Type Selector"=w378:T8, "Specific Arguments"=w380:string)
          n159 = call "Get_array_values_fr_String.vi"("String Value"=w380) -> ("String array"=w381:string[])  [unwired: 1 out]
          n160 = Index Array(array=w381, index=0 ("Index")) -> (element=w377:string)
          n161 = Equal?(x=Multi_run_mode."Auto Calibrate" ("Row Type Selector"), y=w378) -> (x = y?=w374:bool)
          n162 = Equal?(x=w377, y="Concentration") -> (x = y?=w375:bool)
          n163 = Equal?(x=Multi_run_mode."Meas Fast FID Bkgnd" ("Row Type Selector"), y=w378) -> (x = y?=w372:bool)
          n164 = And(x=w374, y=w375) -> (x .and. y?=w373:bool)
        }
        n165 = Or Array Elements(Boolean array=w367) -> (logical OR=w364:bool)
        n166 = Or Array Elements(Boolean array=w366) -> (logical OR=w365:bool)
        n167 = Compound Arithmetic op=AND(invert w364, w365) -> (w362:bool)
        n168 = case shown="True" w362 {
          frame False {
          }
          frame True {
            n169 = One Button Dialog(message="This run automatically calibrates the Fast FID but does not have a Meas Fast FID Bkgnd row" ("format string")) -> ()  [unwired: 2 out]
          }
        }
      }
      frame "First Save Setup file" {
        w385 = -1 ("Currently on Row")
        n170 = case shown="\"Check Multi Run Prog\"" w395 {
          tunnel: [w402 w404 w406 Multi_Run_Case."End" ("Multi Run Case") Multi_Run_Case."End" ("Multi Run Case")] -> w389
          tunnel: w394 -> [w402 w404 w406 _ _]
          tunnel: [w403 w405 w407 w408 w410] -> w388
          frame "Run Multi Run Prog" {
            w403 = FALSE  # Live Traverse Preview?
          }
          frame "Check Multi Run Prog With Live Moves" {
            w405 = TRUE  # Live Traverse Preview?
          }
          frame "Check Multi Run Prog" {
            w407 = FALSE  # Live Traverse Preview?
          }
          frame "Load Command File" {
            w408 = FALSE  # Live Traverse Preview?
          }
          frame "Save Command File" {
            w410 = FALSE  # Live Traverse Preview?
          }
        }
        n171 = local read "Command filename"() -> (w396:path)
        n172 = global write "Trav_pos_global.vi" "Work in Tunnel Coordinates?"("Work in Tunnel Coordinates?") -> ()
        n173 = local write "Currently on Row"(w385) -> ()
        n174 = local write "Last Row Run"(w385) -> ()
        n175 = local read "Jump Bad Positions"() -> (w386:bool)
        n176 = call "Save_Trav_setup.vi"("Work in Tunnel Coordinates?"="Work in Tunnel Coordinates?", "Trav Table"=w397, "Jump Bad Positions"=w386, "Setup filename"=w396) -> ("Trav Table Out"=w398:T6[])  [unwired: 1 out]
        n177 = global write "Meas_global.vi" "Extra Comments"("") -> ()
        n178 = global write "Trav_pos_global.vi" "Live Traverse Preview?"(w388) -> ()
        n179 = local read "Status"() -> (w391:T2)
        n180 = case shown="\"Continue\"" w391 {
          tunnel: [w400 Multi_Run_Case."End" ("Multi Run Case")] -> w390
          tunnel: w389 -> [w400 _]
          frame "Continue" {
          }
          frame "Jump to Next Point", Default {
          }
        }
      }
      frame "Setup Route checking" {
        w415 = string[] []
        n181 = global read "Trav_pos_global.vi" "Work in Tunnel Coordinates?"() -> (w416:T1)
        n182 = for {
          tunnel: w419 -> [w459] mode=indexing
          shift-right: [w450] -> w417
          shift-left: string[] [] -> [w451]
          n183 = Unbundle By Name(w459) -> ("Extra Commands"=w452:string, "Start X"=w456:dbl, "Start Y"=w455:dbl, "Start Z"=w454:dbl)
          n184 = Build Array(w456, w455, w454) -> (w457:dbl[])
          n185 = Not A Number/Path/Refnum?(number/path/refnum=w457) -> (NaN/Path/Refnum?=w458:bool[])
          n186 = Or Array Elements(Boolean array=w458) -> (logical OR=w453:bool)
          n187 = case shown="False" w453 {
            tunnel: w452 -> [w463 _]
            tunnel: w451 -> [w462 w464]
            tunnel: [w461 w464] -> w450
            frame False {
              n188 = call "Which_Trav_Setup.vi"("Extra Command String"=w463) -> ("Traverse Setups"=w460:string[])
              n189 = Build Array (concatenate)(w462, w460) -> (w461:string[])
            }
            frame True {
            }
          }
        }
        n190 = call "Analyse_string_array.vi"("String array"=w417) -> ("Unique strings"=w412:string[])  [unwired: 2 out]
        n191 = for {
          tunnel: w412 -> [w429] mode=indexing
          tunnel: w416 -> [w428]
          shift-right: [w427] -> w413
          shift-left: w415 -> [w426]
          shift-right: [w424] -> w414
          shift-left: w415 -> [w425]
          n192 = stacked-sequence {
            tunnel: w429 -> [w433 w438]
            tunnel: w428 -> [w430 _]
            tunnel: [_ w437] -> w427
            tunnel: w426 -> [_ w436]
            tunnel: w425 -> [_ w435]
            tunnel: [_ w434] -> w424
            frame #0 {
              n193 = call "3D_Traverse_move.vi"("Mode"=Trav_mode."Read traverse position", "Work in Tunnel Coordinates"=w430, "Simulate/Run"=User_Specific_mode."Run VI", "Traverse name"=w433) -> ()  [unwired: 5 in, 7 out]
            }
            frame #1 {
              n194 = global read "DriveConfigGlobal.vi" "Configurations"() -> (w439:T21[])
              n195 = for {
                tunnel: w439 -> [w449] mode=indexing
                tunnel: w438 -> [w446]
                shift-right: [w444] -> w437
                shift-left: w436 -> [w445]
                shift-right: [w440] -> w434
                shift-left: w435 -> [w441]
                i -> [w448]
                n196 = Unbundle By Name(w449) -> ("Channel Properties.Metadata Ch Name"=w443:string)
                n197 = Format Into String(format string="%d", initial string=w446, w448) -> (resulting string=w442:string)  [unwired: 1 in, 1 out]
                n198 = Build Array (concatenate)(w445, w443) -> (w444:string[])
                n199 = Build Array (concatenate)(w441, w442) -> (w440:string[])
              }
            }
          }
        }
        n200 = global write "Trav_pos_global.vi" "ADAM Positions Ch names"(w413) -> ()
        n201 = global write "Route_mapping_global.vi" "Display Mode"("Display Mode") -> ()
        n202 = global write "Trav_pos_global.vi" "Route checking Chs"(w414) -> ()
        n203 = global write "Trav_pos_global.vi" "Traverses to Move"(w412) -> ()
      }
      frame "Initialise Measurement Prog" {
        n204 = for {
          tunnel: w472 -> [w476] mode=indexing
          tunnel: [w475] -> w466 mode=indexing
          n205 = Unbundle By Name(w476) -> ("Meas Setup File"=w475:string)
        }
        n206 = call "Analyse_string_array.vi"("String array"=w466) -> ("Unique strings"=w465:string[])  [unwired: 1 in, 1 out]
        n207 = call "Perform_Meas_Setup.vi"("Simulate/Run"=User_Specific_mode."Check VI only", "String array"=w465) -> ("Continue?"=w467:bool)  [unwired: 1 out]
        n208 = Select(t=w470, s=w467, f=Multi_Run_Case."End" ("Multi Run Case")) -> (s? t:f=w469:T3)
      }
      frame "Input Current Position" {
        n209 = call "Save_ADAM_Table_Locally.vi"() -> ()  [unwired: 12 in]
      }
      frame "Experimental setup control" {
        n210 = global read "Trav_pos_global.vi" "Source Control?"() -> (w484:bool)
        n211 = Equal?(x=w487, y=User_Specific_mode."Run VI" ("Simulate/Run")) -> (x = y?=w486:bool)
        n212 = Or(x=w484, y=w486) -> (x .or. y?=w485:bool)
        n213 = case shown="True" w485 {
          tunnel: w484 -> [_ w491]
          frame False {
          }
          frame True {
            n214 = call "Exp_Setup_Control_remote.vi"("Dispersion?"=w491) -> ()  [unwired: 3 out]
          }
        }
        n215 = global write "Trav_pos_global.vi" "FFID Background"(T6 {"Start X"=nan, "Start Y"=nan, "Start Z"=nan, "End X"=nan, "End Y"=nan, "End Z"=nan, "No. of pts."=0, "Spacing"=enum."Linear", "Filename"=path "", "Tunnel Speed"=nan, "Averaging time (min)"=nan, "Extra Commands"="", "Specific Arguments"="", "Emission Rate (l/min)"=nan, "Trace Gas Concentration (%)"=nan, "Density Ratio"="", "Comments"="", "Row No"=0, "Row Type Selector"=enum."Blank Row", "Completion time"="", "Row Duration (mins)"=nan, "No. of Valid pts."=0, "Meas Setup File"=""} ("FFID Background")) -> ()
      }
      frame "Check source flowrates" {
        n216 = case shown="\"Check VI only\", Default" w492 {
          tunnel: w493 -> [_ w502]
          frame "Check VI only", Default {
            n217 = Get Date/Time In Seconds() -> (seconds since 1Jan1904=w501:timestamp)
            n218 = global write "Trav_pos_global.vi" "Simulation Time"(w501) -> ()
          }
          frame "Run VI" {
            n219 = for {
              tunnel: w502 -> [w503] mode=indexing
              n220 = call "Set_Source.vi"("Source Status"=Client_Source_Status."Using", "Traverse line"=w503, "Simulate/Run"=User_Specific_mode."Check VI only") -> ()  [unwired: 1 in, 6 out]
            }
          }
        }
        n221 = Equal?(x=w492, y=User_Specific_mode."Run VI" ("Simulate/Run")) -> (x = y?=w496:bool)
        n222 = Increment(x=w498) -> (x+1=w494:T3)
        n223 = Select(t=w498, s=w496, f=w494) -> (s? t:f=w495:T3)
      }
      frame "Setup for running mode" {
        n224 = stacked-sequence {
          seq-local: [_ _ _ _ _ w558 _] -> [_ _ _ _ _ _ w576]
          tunnel: w509 -> [_ w533 _ _ w557 _ _]
          tunnel: w508 -> [_ _ _ w552 _ _ _]
          tunnel: [_ _ _ _ w555 _ _] -> w507
          tunnel: [_ _ _ _ _ w558 _] -> w506
          frame #0 {
            n225 = global read "Preference_global.vi" "Rig Setup"() -> (w513:string)
            n226 = Equal?(x=w513, y="EnFlo_Tunnel") -> (x = y?=w512:bool)
            n227 = case shown="True" w512 {
              frame False {
              }
              frame True {
                w518 = "EnFlo_Tunnel:Inlet_Fans:Enable"
                n228 = Build Array(w518) -> (w521:string[])
                n229 = call "Get_Current_Scan_client.vi"("ADAM Ch Names"=w521) -> ("Numerical Values"=w520:dbl[])  [unwired: 3 out]
                n230 = Index Array(array=w520, index=0) -> (element=w517:dbl)
                n231 = Greater?(x=w517, y=0.5) -> (0:w515:bool)
                n232 = case shown="False" w515 {
                  tunnel: w518 -> [w522 _]
                  frame False {
                    n233 = Format Into String(format string="The \"%s\" are not running. Do you want to put them on?", w522) -> (resulting string=w526:string)  [unwired: 2 in, 1 out]
                    n234 = Two Button Dialog(message=w526, 1:"No" ("F button name (\"Cancel\")"), 2:"Yes" ("T button name (\"OK\")")) -> (T button?=w523:bool)
                    n235 = case shown="True" w523 {
                      tunnel: w522 -> [_ w529]
                      frame False {
                      }
                      frame True {
                        n236 = Build Array(w529) -> (w530:string[])
                        n237 = call "ASYNC_Adam_client.vi"("Values"=dbl[] [1.0], "Channel Names"=w530) -> ()  [unwired: 1 in, 2 out]
                      }
                    }
                  }
                  frame True {
                  }
                }
              }
            }
          }
          frame #1 {
            n238 = for {
              tunnel: w533 -> [w537] mode=indexing
              tunnel: [w534] -> w532 mode=indexing
              n239 = Unbundle By Name(w537) -> ("Row Type Selector"=w536:T8)
              n240 = Equal?(x=Multi_run_mode."Synchronize With:" ("Row Type Selector"), y=w536) -> (x = y?=w534:bool)
            }
            n241 = call "Setup_Environment.vi"() -> ()  [unwired: 1 in, 1 out]
            n242 = Or Array Elements(Boolean array=w532) -> (logical OR=w531:bool)
            n243 = case shown="True" w531 {
              frame False {
              }
              frame True {
                n244 = call "Declare_Sync_Client.vi"() -> ()  [unwired: 6 out]
              }
            }
          }
          frame #2 {
            n245 = Open VI Reference(vi path="Display_Trav_Views.vi" ("VI path")) -> (vi reference=w543:refnum<vi>, error out=w542:errorcluster)  [unwired: 1 in, 4 out]
            n246 = global write "Meas_global.vi" "Post Process"(Post_Process."Take New Data" ("Post Process")) -> ()
            n247 = property class="VI"(reference=w543, error in=w542, "Front Panel Window:Open"=FALSE) -> (reference out=w540:refnum<vi>, error out=w539:errorcluster)
            n248 = Close Reference(reference=w540, error in (no error)=w539) -> ()  [unwired: 1 out]
          }
          frame #3 {
            w547 = TRUE  # Start of Multi Run Prog
            w553 = TRUE
            n249 = Get Date/Time In Seconds() -> (seconds since 1Jan1904=w546:timestamp)
            n250 = To Double Precision Float(number=w546) -> (double precision float=w545:dbl)
            n251 = global write "Preference_global.vi" "Unblock Email"(w553) -> ()
            n252 = global write "Preference_global.vi" "Unblock SMS"(w553) -> ()
            n253 = global write "Meas_global.vi" "Start Time of experiment"(w545) -> ()
            n254 = local read "Command filename"() -> (w551:path)
            n255 = Path To String(path=w551) -> (string=w549:string)
            n256 = Concatenate Strings("Commencing a new multi run Prog having the setup filename of :" ("Message"), w549) -> (w548:string)
            n257 = call "Log_Current_row_to_Execute.vi"("Simulate/Run"=w552, "Message"=w548, "Start of Multi Run Prog"=w547) -> ()  [unwired: 2 in, 5 out]
          }
          frame #4 {
            n258 = call "Calc_Remaining_Time.vi"("Currently on Row"=-1, "Table In"=w557) -> ("Estimated Completion time"=w554:string, "Table Out"=w555:T6[])
            n259 = local write "Estimated Completion time"(w554) -> ()
            n260 = global write "Trav_pos_global.vi" "Estimated Completion time"(w554) -> ()
          }
          frame #5 {
            n261 = global read "Trav_pos_global.vi" "Source Control?"() -> (w559:bool)
            n262 = case shown="True" w559 {
              tunnel: [TRUE ("T button?") w564] -> w558
              frame False {
              }
              frame True {
                w565 = "EnFlo_Tunnel:Gas Solenoid:Status"
                n263 = Build Array(w565) -> (w568:string[])
                n264 = call "Get_Current_Scan_client.vi"("ADAM Ch Names"=w568) -> ("Numerical Values"=w567:dbl[])  [unwired: 3 out]
                n265 = Index Array(array=w567, index=0) -> (element=w563:dbl)
                n266 = Greater?(x=w563, y=0.5) -> (0:w561:bool)
                n267 = case shown="False" w561 {
                  tunnel: w565 -> [w574 _]
                  tunnel: [w569 TRUE ("T button?")] -> w564
                  frame False {
                    n268 = Format Into String(format string="The \"%s\" ADAM channel is showing that the blue gas button is not on.", w574) -> (resulting string=w572:string)  [unwired: 2 in, 1 out]
                    n269 = Two Button Dialog(message=w572, 1:"Stop" ("F button name (\"Cancel\")"), 2:"Continue" ("T button name (\"OK\")")) -> (T button?=w569:bool)
                  }
                  frame True {
                  }
                }
              }
            }
          }
          frame #6 {
            n270 = case shown="True" w576 {
              frame False {
              }
              frame True {
                n271 = call "Program_Active_Client.vi"("Mode"=enum16{"Program Active", "Traverse Level State"}."Traverse Level State", "Traverse level State"=Traverse_Level_State."Running") -> ()  [unwired: 1 in, 3 out]
              }
            }
          }
        }
      }
      frame "Skip Blank Rows" {
        n272 = stacked-sequence {
          tunnel: w583 -> [w586 w605]
          tunnel: w580 -> [w584 w601]
          frame #0 {
            n273 = Decrement(x=w586) -> (x-1=w585:i32)
            n274 = while {
              tunnel: w584 -> [w596]
              tunnel: w585 -> [w590]
              stop <- w587 continue-if-true
              n275 = local read "Currently on Row"() -> (w592:i32)
              n276 = Increment(x=w592) -> (x+1=w591:i32)
              n277 = Less?(x=w591, y=w590) -> (x < y?=w589:bool)
              n278 = Index Array(array=w596, index=w591) -> (element=w595:T6)
              n279 = Unbundle By Name(w595) -> ("Row Type Selector"=w594:T8)
              n280 = Equal?(x=Multi_run_mode."Blank Row" ("Row Type Selector"), y=w594) -> (x = y?=w588:bool)
              n281 = case shown="True" w588 {
                tunnel: w591 -> [_ w597]
                frame False {
                }
                frame True {
                  n282 = local write "Currently on Row"(w597) -> ()
                }
              }
              n283 = And(x=w588, y=w589) -> (x .and. y?=w587:bool)
            }
          }
          frame #1 {
            n284 = local read "Currently on Row"() -> (w603:i32)
            n285 = Increment(x=w603) -> (x+1=w602:i32)
            n286 = Index Array(array=w601, index=w602) -> (element=w604:T6)
            n287 = Unbundle By Name(w604) -> ("Row Type Selector"=w600:T8)
            n288 = Equal?(x=Multi_run_mode."Turn Off Row Repeating" ("Row Type Selector"), y=w600) -> (x = y?=w598:bool)
            n289 = while {
              shift-right: [w614] -> _
              shift-left: _ -> [w613]
              tunnel: w605 -> [w610]
              tunnel: w603 -> [w614]
              tunnel: w598 -> [w607]
              stop <- TRUE stop-if-true
              n290 = Decrement(x=w610) -> (x-1=w615:i32)
              n291 = Equal?(x=w614, y=w615) -> (x = y?=w608:bool)
              n292 = Not Equal?(x=w614, y=w613) -> (x != y?=w612:bool)
              n293 = Or(x=w607, y=w608) -> (x .or. y?=w606:bool)
              n294 = And(x=w612, y=w606) -> (x .and. y?=w611:bool)
              n295 = case shown="True" w611 {
                tunnel: w610 -> [_ w616]
                frame False {
                }
                frame True {
                  n296 = Initialize Array(timestamp(0 s since 1904-01-01) ("seconds since 1Jan1904"), w616) -> (w618:timestamp[])
                  n297 = global write "Trav_pos_global.vi" "Row completion times"(w618) -> ()
                }
              }
            }
          }
        }
      }
      frame "Which row to execute next" {
        # "Rep?"
        # "Repeat\nRow"
        n298 = local read "Currently on Row"() -> (w619:i32)
        n299 = stacked-sequence {
          seq-local: [_ w658 _] -> [_ _ w694]
          seq-local: [_ w657 _] -> [_ _ w695]
          seq-local: [w628 _ _] -> [_ w656 _]
          seq-local: [_ w653 _] -> [_ _ w688]
          tunnel: [w633 _ _] -> w625
          tunnel: w624 -> [w633 w660 w702]
          tunnel: w623 -> [_ _ w700]
          tunnel: w622 -> [_ w655 w701]
          tunnel: [_ _ w697] -> w621
          tunnel: w620 -> [_ _ w696]
          tunnel: w619 -> [w630 w652 w687]
          frame #0 {
            n300 = Array Size(array=w633) -> (size(s)=w632:i32)
            n301 = Decrement(x=w632) -> (x-1=w631:i32)
            n302 = Increment(x=w630) -> (x+1=w629:i32)
            n303 = while {
              tunnel: w629 -> [w637]
              tunnel: w633 -> [w649] mode=indexing
              tunnel: Multi_run_mode."Turn Off Row Repeating" ("Row Type Selector") -> [w648]
              tunnel: w631 -> [w644]
              tunnel: [w639] -> w628
              i -> [w641]
              stop <- w647 continue-if-true
              n304 = Less?(x=w641, y=w637) -> (x < y?=w642:bool)
              n305 = Unbundle By Name(w649) -> ("Row Type Selector"=w646:T8)
              n306 = Less?(x=w641, y=w644) -> (x < y?=w643:bool)
              n307 = Equal?(x=w641, y=w637) -> (x = y?=w638:bool)
              n308 = Equal?(x=w648, y=w646) -> (x = y?=w640:bool)
              n309 = case shown="True" w640 {
                tunnel: [TRUE w651] -> w639
                tunnel: w638 -> [_ w651]
                frame False {
                }
                frame True {
                }
              }
              n310 = Not(x=w640) -> (.not. x?=w645:bool)
              n311 = Compound Arithmetic op=AND(w645, w642, w643) -> (w647:bool)
            }
            n312 = global write "Trav_pos_global.vi" "Currently on point"(0 ("Currently on point")) -> ()
            n313 = global write "Trav_pos_global.vi" "Paused During Row?"(FALSE ("Paused During Row?")) -> ()
            n314 = global write "Trav_pos_global.vi" "Repeat Rows?"(w628) -> ()
          }
          frame #1 {
            n315 = global read "Trav_pos_global.vi" "Row completion times"() -> (w659:timestamp[])
            n316 = global read "Extra_Commands_Global.vi" "Minutes Before Repeating Row"() -> (w654:string)
            n317 = case shown="\"Run VI\"" w655 {
              tunnel: [w661 w662] -> w653
              frame "Check VI only" {
                n318 = global read "Trav_pos_global.vi" "Simulation Time"() -> (w661:timestamp)
              }
              frame "Run VI" {
                n319 = Get Date/Time In Seconds() -> (seconds since 1Jan1904=w662:timestamp)
                n320 = global write "Trav_pos_global.vi" "Simulation Time"(w662) -> ()
              }
            }
            n321 = while {
              tunnel: w660 -> [w672] mode=indexing
              tunnel: w659 -> [w675]
              tunnel: w653 -> [w674]
              tunnel: [w665] -> w658
              tunnel: [w664] -> w657
              tunnel: w656 -> [w668]
              tunnel: w652 -> [w666]
              tunnel: w654 -> [w663]
              i -> [w664]
              stop <- w671 continue-if-true
              n322 = Unbundle By Name(w672) -> ("Extra Commands"=w676:string)
              n323 = call "Extra_Commands.vi"("String to Search"=w676, "Command"=w663) -> ("Numeric Value"=w673:dbl, "Command Found"=w669:bool)  [unwired: 1 in, 3 out]
              n324 = And(x=w668, y=w669) -> (x .and. y?=w667:bool)
              n325 = case shown="True" w667 {
                tunnel: w675 -> [_ w682]
                tunnel: w674 -> [_ w683]
                tunnel: w664 -> [_ w681]
                tunnel: w673 -> [_ w679]
                tunnel: [FALSE w678] -> w665
                frame False {
                }
                frame True {
                  n326 = Index Array(array=w682, index=w681) -> (element=w684:timestamp)
                  n327 = Subtract(x=w683, y=w684) -> (x-y=w685:dbl)
                  n328 = Divide(x=w685, y=60.0) -> (x/y=w680:dbl)
                  n329 = Greater?(x=w680, y=w679) -> (0:w678:bool)
                }
              }
              n330 = Less?(x=w664, y=w666) -> (x < y?=w670:bool)
              n331 = Compound Arithmetic op=AND(invert w665, w670) -> (w671:bool)
            }
          }
          frame #2 {
            n332 = Not Equal?(x=w687, y=w695) -> (x != y?=w693:bool)
            n333 = And(x=w694, y=w693) -> (x .and. y?=w692:bool)
            n334 = case shown="False" w692 {
              tunnel: w695 -> [_ w728]
              tunnel: w687 -> [w724 w730]
              tunnel: [w723 w729] -> w698
              tunnel: [w723 w728] -> w689
              tunnel: w700 -> [w726 _]
              tunnel: [w722 TRUE] -> w699
              frame False {
                n335 = Increment(x=w724) -> (x+1=w725:i32)
                n336 = Greater?(x=w726, y=w725) -> (0:w722:bool)
                n337 = Select(t=w725, s=w722, f=w724) -> (s? t:f=w723:i32)
              }
              frame True {
                n338 = Greater?(x=w730, y=w728) -> (0:w731:bool)
                n339 = Select(t=w730, s=w731, f=w728) -> (s? t:f=w729:i32)
              }
            }
            n340 = global read "Trav_pos_global.vi" "Row completion times"() -> (w691:timestamp[])
            n341 = case shown="True" w699 {
              tunnel: w689 -> [_ w710]
              tunnel: w702 -> [_ w716]
              tunnel: w701 -> [w704 w708]
              tunnel: w698 -> [_ w714]
              tunnel: [w703 w713] -> w697
              tunnel: w696 -> [_ w713]
              frame False {
                n342 = case shown="\"Run VI\"" w704 {
                  tunnel: [Multi_Run_Case."Show jumped positions" ("Multi Run Case") Multi_Run_Case."Shut down source etc" ("Multi Run Case")] -> w703
                  frame "Check VI only" {
                  }
                  frame "Run VI" {
                  }
                }
              }
              frame True {
                n343 = Index Array(array=w716, index=w710) -> (element=w712:T6)
                n344 = Bundle By Name(cluster=w712, "Row No"=w710) -> (w711:T6)
                n345 = global write "Trav_pos_global.vi" "Meas Setup Number"(0 ("Meas Setup Number")) -> ()
                n346 = Build Array(w714) -> (w715:i32[])
                n347 = case shown="\"Run VI\"" w708 {
                  tunnel: w708 -> [_ w720]
                  tunnel: w711 -> [w717 w719]
                  tunnel: [w717 w718] -> w707
                  frame "Check VI only" {
                  }
                  frame "Run VI" {
                    n348 = call "Log_Current_row_to_Execute.vi"("Simulate/Run"=w720, "Start of Multi Run Prog"=FALSE, "Traverse line in"=w719) -> ("Traverse line Out"=w718:T6)  [unwired: 2 in, 4 out]
                  }
                }
                n349 = property on="Table" class="Arr (strict)"("Index Values"=w715) -> ()  [unwired: 2 in, 2 out]
                n350 = global write "Trav_pos_global.vi" "Current Row"(w707) -> ()
                "Currently on Row" <- w714
              }
            }
            n351 = Replace Array Subset(array=w691, new element=w688, index=w689) -> (w690:timestamp[])
            n352 = global write "Trav_pos_global.vi" "Row completion times"(w690) -> ()
          }
        }
      }
      frame "Evaluate IF Statement" {
        n353 = global read "Trav_pos_global.vi" "Current Row"() -> (w736:T6)
        n354 = Unbundle By Name(w736) -> ("Extra Commands"=w739:string)
        n355 = global read "Extra_Commands_Global.vi" "If Command"() -> (w742:string)
        n356 = call "Extra_Commands.vi"("String to Search"=w739, "Command"=w742) -> ("String Value"=w741:string, "Command Found"=w733:bool)  [unwired: 1 in, 3 out]
        n357 = Equal?(x=w737, y=User_Specific_mode."Run VI" ("Simulate/Run")) -> (x = y?=w732:bool)
        n358 = And(x=w733, y=w732) -> (x .and. y?=w734:bool)
        n359 = case shown="True" w734 {
          tunnel: w741 -> [_ w752]
          tunnel: [w748 w751] -> w735
          frame False {
            w748 = TRUE  # Execute Row?
          }
          frame True {
            n360 = call "Get_array_values_fr_String.vi"("String Value"=w752) -> ("Numeric Array"=w750:dbl[], "String array"=w749:string[])
            n361 = Index Array(array=w749, index=0 ("Index")) -> (element=w753:string)
            n362 = case shown="\"Global Value Between\"" w753 {
              tunnel: w752 -> [w758 _ _ _]
              tunnel: [w757 w759 w769 TRUE ("Execute Row?")] -> w751
              tunnel: w750 -> [_ w765 w783 _]
              tunnel: w749 -> [_ _ w777 _]
              frame "Time Between" {
                n363 = Get Date/Time In Seconds() -> (seconds since 1Jan1904=w755:timestamp)
                n364 = To Double Precision Float(number=w755) -> (double precision float=w756:dbl)
                n365 = call "If_Time_arguments.vi"("seconds since 1Jan1904"=w756, "String Value"=w758) -> ("Execute Row?"=w757:bool)  [unwired: 2 out]
              }
              frame "Global Value Between" {
                n366 = global read "Extra_Commands_Global.vi" "If command global value"() -> (w760:dbl)
                n367 = Index Array(array=w765, index=1 ("Index")) -> (element=w763:dbl)
                n368 = Index Array(array=w765, index=2 ("Index")) -> (element=w764:dbl)
                n369 = Max & Min(x=w763, y=w764) -> (max(x,y)=w762:dbl, min(x,y)=w761:dbl)
                n370 = In Range and Coerce(upper limit=w762, x=w760, lower limit=w761) -> (In Range?=w759:bool)  [unwired: 1 out]
              }
              frame "ADAM Channel Between" {
                n371 = Index Array(array=w777, index=1 ("Index")) -> (element=w776:string)
                n372 = Build Array(w776) -> (w775:string[])
                n373 = Index Array(array=w783, index=2 ("Index")) -> (element=w781:dbl)
                n374 = Index Array(array=w783, index=3 ("Index")) -> (element=w782:dbl)
                n375 = Max & Min(x=w781, y=w782) -> (max(x,y)=w780:dbl, min(x,y)=w779:dbl)
                n376 = call "Get_Current_Scan_client.vi"("ADAM Ch Names"=w775) -> ("Numerical Values"=w773:dbl[])  [unwired: 3 out]
                n377 = Index Array(array=w773, index=0 ("Index")) -> (element=w772:dbl)
                n378 = In Range and Coerce(upper limit=w780, x=w772, lower limit=w779) -> (In Range?=w770:bool)  [unwired: 1 out]
                n379 = Not A Number/Path/Refnum?(number/path/refnum=w772) -> (NaN/Path/Refnum?=w771:bool)
                n380 = Select(t=TRUE, s=w771, f=w770) -> (s? t:f=w769:bool)
              }
              frame "No Match", Default {
              }
            }
          }
        }
        n381 = Select(t=w745, s=w735, f=Multi_Run_Case."Calculate Row TIme" ("Multi Run Case")) -> (s? t:f=w744:T3)
      }
      frame "Perform Measurement Setup" {
        n382 = global read "Trav_pos_global.vi" "Current Row"() -> (w789:T6)
        n383 = case shown="\"Run VI\"" w788 {
          tunnel: w789 -> [_ w794]
          tunnel: w788 -> [_ w793]
          frame "Check VI only" {
          }
          frame "Run VI" {
            n384 = stacked-sequence {
              tunnel: w794 -> [w797 _]
              tunnel: w793 -> [w795 _]
              frame #0 {
                n385 = Unbundle By Name(w797) -> ("Extra Commands"=w796:string)
                n386 = call "Pause_for_server_ch_val.vi"("Extra command string"=w796, "Simulate/Run"=w795) -> ()  [unwired: 2 out]
              }
              frame #1 {
                n387 = Get Date/Time In Seconds() -> (seconds since 1Jan1904=w798:timestamp)
                n388 = To Double Precision Float(number=w798) -> (double precision float=w799:dbl)
                n389 = global write "Trav_pos_global.vi" "Start of Row time (Sec)"(w799) -> ()
              }
            }
          }
        }
      }
      frame "Set Measurement Conditions" {
        w805 = TRUE  # Row Completed
        w804 = FALSE  # Row Completed
        n390 = global read "Trav_pos_global.vi" "Current Row"() -> (w802:T6)
        n391 = Unbundle By Name(w802) -> ("Row Type Selector"=w807:T8)
        n392 = case shown="\"Send Message\"" w807 {
          tunnel: [TRUE FALSE TRUE TRUE TRUE TRUE FALSE TRUE FALSE w856 FALSE FALSE FALSE] -> w812
          tunnel: w802 -> [w820 w823 w826 w829 w832 w835 w838 w841 w850 w855 w880 w883 w886]
          tunnel: [w820 w823 w826 w829 w832 w835 w838 w841 w849 w854 w880 w883 w886] -> w808
          tunnel: [w819 w822 w825 w828 w831 w834 w837 w840 w845 w852 w879 w882 w885] -> w806
          tunnel: w805 -> [w819 _ w825 w828 w831 _ _ _ _ w852 w879 w882 w885]
          tunnel: w804 -> [_ w822 _ _ _ w834 w837 w840 w845 _ _ _ _]
          tunnel: w801 -> [_ _ _ _ _ _ _ _ _ w853 _ _ _]
          frame "Move Traverse Only" {
          }
          frame "Check Beam Power" {
          }
          frame "Set Tunnel Speed Only" {
          }
          frame "Set Source Only" {
          }
          frame "Set Measurement Conditions" {
          }
          frame "Single Measurement" {
          }
          frame "Vertical Profile", Default {
          }
          frame "Scanning Valve Measurement" {
          }
          frame "Run VI Named:" {
            n393 = global read "Extra_Commands_Global.vi" "Skip Source Demand"() -> (w848:string)
            n394 = global read "Extra_Commands_Global.vi" "Establish Exp Conditions (s)"() -> (w844:string)
            n395 = Unbundle By Name(w850) -> ("Extra Commands"=w847:string)
            n396 = Concatenate Strings(w844, " = 0" ("Substring"), w848, w847) -> (w846:string)
            n397 = Bundle By Name(cluster=w850, "Extra Commands"=w846) -> (w849:T6)
          }
          frame "Send Message" {
            n398 = stacked-sequence {
              seq-local: [w857 _ _ _] -> [_ w865 _ _]
              tunnel: [_ _ _ FALSE] -> w856
              tunnel: w855 -> [_ w867 w873 w876]
              tunnel: [_ _ _ w876] -> w854
              tunnel: w853 -> [w858 _ _ _]
              frame #0 {
                n399 = Equal?(x=User_Specific_mode."Run VI" ("Simulate/Run"), y=w858) -> (x = y?=w857:bool)
              }
              frame #1 {
                n400 = Unbundle By Name(w867) -> ("Specific Arguments"=w861:string, "Comments"=w862:string, "Filename"=w864:path)
                n401 = Concatenate Strings(w861, w862) -> (w860:string)
                n402 = Build Array(w864) -> (w863:path[])
                n403 = case shown="True" w865 {
                  tunnel: "Message" ("Error Type") -> [_ w870]
                  tunnel: w860 -> [_ w869]
                  tunnel: w863 -> [_ w868]
                  frame False {
                  }
                  frame True {
                    n404 = call "Email_Text_Files.vi"("Filenames"=w868, "message"=w869, "subject ([No Subject])"=w870) -> ()
                  }
                }
              }
              frame #2 {
                n405 = global read "Extra_Commands_Global.vi" "Establish Exp Conditions (s)"() -> (w875:string)
                n406 = Unbundle By Name(w873) -> ("Extra Commands"=w874:string)
                n407 = call "Extra_Commands.vi"("String to Search"=w874, "Command"=w875) -> ("Numeric Value"=w871:dbl)  [unwired: 1 in, 4 out]
                n408 = call "Wait_Seconds_with_display.vi"("Message"="In Send Message Row", "Seconds to wait"=w871) -> ()  [unwired: 2 out]
              }
              frame #3 {
              }
            }
          }
          frame "Fall Back to this Row" {
          }
          frame "Turn Off Row Repeating" {
          }
          frame "Blank Row" {
          }
        }
        n409 = case shown="True" w812 {
          tunnel: w808 -> [_ w888]
          tunnel: w801 -> [_ w892]
          tunnel: [Multi_Run_Status."Continue" ("Status") w889] -> w800
          frame False {
          }
          frame True {
            w891 = 1  # Currently on Point
            n410 = call "Program_Active.vi"() -> ()  [unwired: 1 in]
            n411 = call "Set_Measurement_Conditions.vi"("Simulate/Run"=w892, "Currently on Point"=w891, "Traverse line"=w888) -> ("Status Cluster"=w890:T24)  [unwired: 2 out]
            n412 = Unbundle By Name(w890) -> ("Status"=w889:T2)
          }
        }
        n413 = case shown="\"Continue\"" w800 {
          tunnel: [w816 Multi_Run_Case."Calculate Row TIme" ("Multi Run Case")] -> w811
          tunnel: w810 -> [w817 _]
          tunnel: w806 -> [w814 _]
          frame "Continue" {
            n414 = Select(t=Multi_Run_Case."Calculate Row TIme" ("Multi Run Case"), s=w814, f=w817) -> (s? t:f=w816:T3)
          }
          frame "Jump to Next Point", Default {
          }
        }
        n415 = local write "Status"(w800) -> ()
      }
      frame "Execute Row" {
        n416 = global read "Trav_pos_global.vi" "Current Row"() -> (w894:T6)
        n417 = stacked-sequence {
          tunnel: w895 -> [w899 w910 w912]
          tunnel: w894 -> [w900 w907 w911]
          frame #0 {
            n418 = case shown="\"Check VI only\"" w899 {
              tunnel: w900 -> [w903 _]
              tunnel: w899 -> [w902 _]
              frame "Check VI only" {
                n419 = Unbundle By Name(w903) -> ("Extra Commands"=w904:string, "Row No"=w906:i32, "Meas Setup File"=w901:string)
                n420 = call "Skip_If Sd_Error_Below.vi"("String to Search"=w904, "Simulate/Run"=w902, "Measurement setup Applied?"=TRUE, "Row Number"=w906, "Measurement Setup File"=w901) -> ()  [unwired: 5 out]
              }
              frame "Run VI" {
              }
            }
          }
          frame #1 {
            n421 = call "Execute_Row.vi"("Simulate/Run"=w910, "Traverse line"=w907) -> ("Status"=w909:T2, "Traverse line out"=w908:T6)  [unwired: 2 out]
            n422 = local write "Status"(w909) -> ()
            n423 = global write "Trav_pos_global.vi" "Current Row"(w908) -> ()
          }
          frame #2 {
            w915 = FALSE  # Empty list
            n424 = call "Remember_RD_Folders.vi"("Empty list"=w915) -> ("List of Folders"=w914:path[])  [unwired: 1 in]
            n425 = for {
              tunnel: w911 -> [w920]
              tunnel: w914 -> [w919] mode=indexing
              tunnel: "Muti_Run_Log.xls" ("name or relative path") -> [w917]
              tunnel: w912 -> [w916]
              n426 = Build Path(base path=w919, name or relative path=w917) -> (appended path=w918:path)
              n427 = call "Log_Current_row_to_Execute.vi"("Simulate/Run"=w916, "Start of Multi Run Prog"=FALSE, "Traverse line in"=w920, "Multi Run Log File"=w918) -> ()  [unwired: 1 in, 5 out]
            }
          }
        }
      }
      frame "Calculate Row TIme" {
        n428 = global read "Trav_pos_global.vi" "Paused During Row?"() -> (w925:bool)
        n429 = local read "Status"() -> (w928:T2)
        n430 = global read "Trav_pos_global.vi" "Current Row"() -> (w924:T6)
        n431 = Equal?(x=w928, y=Multi_Run_Status."Continue" ("Status")) -> (x = y?=w927:bool)
        n432 = Equal?(x=w930, y=User_Specific_mode."Run VI" ("Simulate/Run")) -> (x = y?=w926:bool)
        n433 = Compound Arithmetic op=AND(w927, w926, invert w925) -> (w923:bool)
        n434 = case shown="False" w923 {
          tunnel: w924 -> [w943 w954]
          frame False {
            n435 = global read "Trav_pos_global.vi" "Simulation Time"() -> (w944:timestamp)
            n436 = To Double Precision Float(number=w944) -> (double precision float=w938:dbl)
            n437 = call "Calculate_Row_Time.vi"("Row Start Time (Sec Since 1904)"=w938, "Multi Run Row"=w943) -> ("Scalable Time (Sec)"=w941:dbl, "Fixed Time (Sec)"=w939:dbl)
            n438 = call "Overhead_Factor.vi"("Mode"=Overhead."Read Current Overhead") -> ("Current Overhead Factor"=w942:dbl)  [unwired: 3 in]
            n439 = Multiply(x=w942, y=w941) -> (x*y=w940:dbl)
            n440 = Add(x=w939, y=w940) -> (x+y=w935:dbl)
            n441 = global write "Trav_pos_global.vi" "Start of Row time (Sec)"(w935) -> ()
            n442 = Add(x=w938, y=w935) -> (x+y=w937:dbl)
            n443 = To Time Stamp(1:w937) -> (0:w936:timestamp)
            n444 = global write "Trav_pos_global.vi" "Simulation Time"(w936) -> ()
          }
          frame True {
            n445 = global read "Trav_pos_global.vi" "Start of Row time (Sec)"() -> (w952:dbl)
            n446 = Get Date/Time In Seconds() -> (seconds since 1Jan1904=w947:timestamp)
            n447 = To Double Precision Float(number=w947) -> (double precision float=w946:dbl)
            n448 = call "Calculate_Row_Time.vi"("Row Start Time (Sec Since 1904)"=w952, "Multi Run Row"=w954) -> ("Scalable Time (Sec)"=w948:dbl, "Fixed Time (Sec)"=w950:dbl)
            n449 = Subtract(x=w946, y=w952) -> (x-y=w951:dbl)
            n450 = Subtract(x=w951, y=w950) -> (x-y=w949:dbl)
            n451 = call "Overhead_Factor.vi"("Sum of Ideal times (Sec)"=w948, "Sum of Actual times (Sec)"=w949, "Mode"=Overhead."Update total times") -> ()  [unwired: 1 in, 1 out]
          }
        }
      }
      frame "Update time estimate" {
        n452 = global read "Trav_pos_global.vi" "Current Row"() -> (w958:T6)
        n453 = Unbundle By Name(w958) -> ("Row No"=w956:i32)
        n454 = local read "Currently on Row"() -> (w957:i32)
        n455 = Equal?(x=w956, y=w957) -> (x = y?=w955:bool)
        n456 = case shown="\"Run VI\"" w961 {
          tunnel: w964 -> [w972 w995]
          tunnel: [w971 w991] -> w963
          tunnel: w960 -> [_ w997]
          tunnel: [w970 w996] -> w959
          tunnel: w957 -> [w968 w990]
          tunnel: w958 -> [w969 w994]
          tunnel: w955 -> [w967 w993]
          frame "Check VI only" {
            n457 = global read "Trav_pos_global.vi" "Simulation Time"() -> (w974:timestamp)
            n458 = To Double Precision Float(number=w974) -> (double precision float=w973:dbl)
            n459 = call "Sec_to_date_filename.vi"("seconds"=w973) -> ("Day"=w976:string, "Time"=w975:string)  [unwired: 2 out]
            n460 = Concatenate Strings(w975, "  " ("Substring"), w976) -> (w970:string)
            n461 = case shown="True" w967 {
              tunnel: w968 -> [_ w987]
              tunnel: w972 -> [w978 w986]
              tunnel: [w978 w984] -> w971
              tunnel: w970 -> [_ w983]
              tunnel: w969 -> [_ w982]
              frame False {
              }
              frame True {
                n462 = global read "Trav_pos_global.vi" "Start of Row time (Sec)"() -> (w981:dbl)
                n463 = Divide(x=w981, y=60.0) -> (x/y=w979:dbl)
                n464 = Bundle By Name(cluster=w982, "Completion time"=w983, "Row Duration (mins)"=w979) -> (w985:T6)
                n465 = Replace Array Subset(array=w986, new element=w985, index=w987) -> (w984:T6[])
              }
            }
          }
          frame "Run VI" {
            n466 = case shown="True" w993 {
              tunnel: w990 -> [_ w1004]
              tunnel: w995 -> [w1000 w1003]
              tunnel: w994 -> [_ w1002]
              tunnel: [w1000 w1001] -> w992
              frame False {
              }
              frame True {
                n467 = Replace Array Subset(array=w1003, new element=w1002, index=w1004) -> (w1001:T6[])
              }
            }
            n468 = call "Calc_Remaining_Time.vi"("Currently on Row"=w990, "Table In"=w992) -> ("Table Out"=w991:T6[])  [unwired: 1 out]
            n469 = Decrement(x=w997) -> (x-1=w999:i32)
            n470 = Index Array(array=w991, index=w999) -> (element=w998:T6)
            n471 = Unbundle By Name(w998) -> ("Completion time"=w996:string)
            n472 = call "Program_Active_Client.vi"("Mode"=enum16{"Program Active", "Traverse Level State"}."Traverse Level State", "Traverse level State"=Traverse_Level_State."Running") -> ()  [unwired: 1 in, 3 out]
          }
        }
        "Estimated Completion time" <- w959
        n473 = global write "Trav_pos_global.vi" "Estimated Completion time"(w959) -> ()
      }
      frame "Pause Multi Run Program" {
        n474 = while {
          tunnel: "Pause" -> [w1016]
          tunnel: [w1019] -> w1011
          tunnel: w1010 -> [w1018]
          tunnel: w1008 -> [w1017]
          shift-right: [w1016] -> _
          shift-left: _ -> [w1015]
          stop <- TRUE stop-if-true
          n475 = case shown="True" w1016 {
            tunnel: [w1020 w1025] -> w1019
            tunnel: w1018 -> [w1020 w1023]
            tunnel: w1017 -> [_ w1024]
            tunnel: w1016 -> [_ w1022]
            tunnel: w1015 -> [_ w1021]
            frame False {
            }
            frame True {
              n476 = stacked-sequence {
                tunnel: w1023 -> [_ _ _ _ w1040]
                tunnel: [_ _ _ _ w1041] -> w1025
                tunnel: w1024 -> [w1027 _ _ _ _]
                tunnel: w1022 -> [_ _ _ w1036 _]
                tunnel: w1021 -> [_ _ _ w1035 _]
                frame #0 {
                  n477 = Quotient & Remainder(x=w1027, y=15) -> (x-y*floor(x/y)=w1026:i32)  [unwired: 1 out]
                  n478 = case shown="0" w1026 {
                    frame 0 {
                      n479 = Current VI's Path() -> (path=w1029:path)
                      n480 = call "Bring_to_front.vi"("path"=w1029) -> ()
                    }
                    frame 1, Default {
                    }
                  }
                }
                frame #1 {
                  n481 = global write "Trav_pos_global.vi" "Paused During Row?"(TRUE ("Paused During Row?")) -> ()
                  "Pause message" <- "Multi Run Program Paused!!!!" ("Pause message")
                }
                frame #2 {
                  n482 = property on="Pause message" class="Str"("Visible"=TRUE) -> ()  [unwired: 2 in, 2 out]
                  n483 = Wait Until Next ms Multiple(millisecond multiple=u32 1500) -> ()  [unwired: 1 out]
                }
                frame #3 {
                  n484 = Compound Arithmetic op=AND(w1036, invert w1035) -> (w1034:bool)
                  n485 = case shown="True" w1034 {
                    frame False {
                    }
                    frame True {
                      n486 = call "Program_Active_Client.vi"("Mode"=enum16{"Program Active", "Traverse Level State"}."Program Active", "Time till next contact (Sec)"=12000.0, "Traverse level State"=Traverse_Level_State."Running") -> ()  [unwired: 3 out]
                    }
                  }
                }
                frame #4 {
                  n487 = property on="Pause message" class="Str"("Visible"=FALSE) -> ()  [unwired: 2 in, 2 out]
                  n488 = Wait Until Next ms Multiple(millisecond multiple=u32 1500) -> ()  [unwired: 1 out]
                  n489 = Decrement(x=w1040) -> (x-1=w1041:T3)
                }
              }
            }
          }
        }
        n490 = call "Overhead_Factor.vi"("Mode"=Overhead."Read Current Overhead") -> ("Current Overhead Factor"=→"Current Overhead Factor":dbl)  [unwired: 3 in]
      }
      frame "Do Another Row?" {
        w1058 = Multi_Run_Status."Terminate Run" ("Status")
        n491 = case shown="False" "Stop after Repeats" {
          tunnel: [w1079 w1080] -> w1052
          tunnel: w1048 -> [_ w1081]
          frame False {
            n492 = local read "Currently on Row"() -> (w1079:i32)
            n493 = Increment(x=w1079) -> (x+1=→"Last Row Run":i32)
          }
          frame True {
            n494 = Decrement(x=w1081) -> (x-1=w1080:i32)
            n495 = local write "Currently on Row"(w1080) -> ()
          }
        }
        n496 = global read "Preference_global.vi" "Server Comms"() -> (w1047:T25)
        n497 = case shown="\"Server Link Healthy\"" w1047 {
          tunnel: [w1067 TRUE] -> w1046
          frame "Server Link Healthy" {
            n498 = Build Array("EnFlo Lab:Emergency_Stop:Happy") -> (w1070:string[])
            n499 = call "Get_Current_Scan_client.vi"("ADAM Ch Names"=w1070) -> ("Numerical Values"=w1072:dbl[])  [unwired: 1 in, 2 out]
            n500 = Index Array(array=w1072) -> (element=w1068:dbl)  [unwired: 1 in]
            n501 = Not A Number/Path/Refnum?(number/path/refnum=w1068) -> (NaN/Path/Refnum?=w1069:bool)
            n502 = case shown="False" w1069 {
              tunnel: w1068 -> [w1075 _]
              tunnel: [w1073 TRUE] -> w1067
              frame False {
                n503 = Greater?(x=w1075, y=0.5) -> (0:w1073:bool)
              }
              frame True {
              }
            }
          }
          frame "Do Not Link To Server" {
          }
        }
        n504 = case shown="True" "stop" {
          tunnel: [w1082 w1083] -> w1059
          tunnel: w1058 -> [_ w1083]
          frame False {
            n505 = local read "Status"() -> (w1082:T2)
          }
          frame True {
            n506 = local write "Status"(w1083) -> ()
          }
        }
        n507 = Not Equal?(x=w1059, y=w1058) -> (x != y?=w1057:bool)
        n508 = Increment(x=w1052) -> (x+1=w1051:i32)
        n509 = Index Array(array=w1053, index=w1051) -> (element=w1050:T6)
        n510 = Unbundle By Name(w1050) -> ("Row Type Selector"=w1056:T8)
        n511 = Equal?(x=w1056, y=Multi_run_mode."Turn Off Row Repeating" ("Row Type Selector")) -> (x = y?=w1054:bool)
        n512 = case shown="False" w1057 {
          tunnel: [w1084 w1088] -> w1044
          tunnel: w1062 -> [w1085 _]
          tunnel: w1053 -> [_ _]
          tunnel: w1059 -> [_ w1089]
          tunnel: w1054 -> [_ _]
          frame False {
            n513 = case shown="\"Run VI\"" w1085 {
              tunnel: [Multi_Run_Case."Show jumped positions" ("Multi Run Case") Multi_Run_Case."Shut down source etc" ("Multi Run Case")] -> w1084
              frame "Check VI only" {
              }
              frame "Run VI" {
              }
            }
          }
          frame True {
            n514 = case shown="\"Jump To Fall Back\"" w1089 {
              tunnel: [Multi_Run_Case."Skip Blank Rows" ("Multi Run Case") Multi_Run_Case."Find Next Fall Back Row" ("Multi Run Case")] -> w1088
              frame "Continue", Default {
              }
              frame "Jump To Fall Back" {
              }
            }
          }
        }
        n515 = case shown="False" w1046 {
          tunnel: [Multi_Run_Case."Shut down source etc" ("Multi Run Case") w1066] -> w1045
          tunnel: w1044 -> [_ w1066]
          frame False {
            n516 = local write "Status"(Multi_Run_Status."Terminate Run" ("Status")) -> ()
          }
          frame True {
          }
        }
      }
      frame "Find Next Fall Back Row" {
        n517 = local read "Currently on Row"() -> (w1093:i32)
        n518 = Increment(x=w1093) -> (x+1=w1092:i32)
        n519 = Index Array(array=w1101, index=w1093) -> (element=w1102:T6)
        n520 = Array Size(array=w1101) -> (size(s)=w1100:i32)
        n521 = Unbundle By Name(w1102) -> ("Row Type Selector"=w1096:T8)
        n522 = Greater?(x=w1100, y=w1092) -> (0:w1099:bool)
        n523 = Equal?(x=w1096, y=Multi_run_mode."Fall Back to this Row" ("Mode")) -> (x = y?=w1094:bool)
        n524 = case shown="True" w1099 {
          tunnel: [Multi_Run_Case."Skip Blank Rows" ("Multi Run Case") w1109] -> w1098
          tunnel: w1094 -> [_ w1105]
          tunnel: w1093 -> [_ w1106]
          frame False {
          }
          frame True {
            n525 = case shown="False" w1105 {
              tunnel: w1106 -> [w1111 _]
              frame False {
                n526 = Increment(x=w1111) -> (x+1=w1110:i32)
                n527 = local write "Currently on Row"(w1110) -> ()
              }
              frame True {
              }
            }
            n528 = Select(t=Multi_Run_Case."Skip Blank Rows" ("Multi Run Case"), s=w1105, f=Multi_Run_Case."Find Next Fall Back Row" ("Multi Run Case")) -> (s? t:f=w1109:T3)
          }
        }
      }
      frame "Shut down source etc" {
        n529 = for {
          tunnel: w1131 -> [w1149] mode=indexing
          tunnel: Multi_run_mode."Synchronize With:" ("Mode") -> [w1147]
          tunnel: [w1146] -> w1133 mode=indexing
          n530 = Unbundle By Name(w1149) -> ("Row Type Selector"=w1148:T8)
          n531 = Equal?(x=w1148, y=w1147) -> (x = y?=w1146:bool)
        }
        n532 = call "Overhead_Factor.vi"("Mode"=Overhead."Re Scale totals to 3 hrs") -> ()  [unwired: 3 in, 1 out]
        n533 = local read "Status"() -> (w1119:T2)
        n534 = call "Set_Source.vi"("Source Status"=Client_Source_Status."Not Using", "Simulate/Run"=w1122) -> ("Status Cluster"=w1123:T24)  [unwired: 2 in, 5 out]
        n535 = call "Program_Active_Client.vi"("Mode"=enum16{"Program Active", "Traverse Level State"}."Traverse Level State", "Traverse level State"=Traverse_Level_State."Complete") -> ()  [unwired: 1 in, 3 out]
        n536 = global read "Meas_global.vi" "Start Time of experiment"() -> (w1129:dbl)
        n537 = Equal?(x=w1119, y=Multi_Run_Status."Terminate Run" ("Status")) -> (x = y?=w1117:bool)
        n538 = call "Prog_Status_Handler.vi"("Status Cluster"=w1123, "Simulate/Run"=w1122) -> ()  [unwired: 2 out]
        n539 = Or Array Elements(Boolean array=w1133) -> (logical OR=w1120:bool)
        n540 = Get Date/Time In Seconds() -> (seconds since 1Jan1904=w1112:timestamp)
        n541 = Compound Arithmetic op=AND(w1120, invert w1117) -> (w1121:bool)
        n542 = To Double Precision Float(number=w1112) -> (double precision float=w1130:dbl)
        n543 = case shown="True" w1121 {
          frame False {
          }
          frame True {
            n544 = global read "Preference_global.vi" "Rig Setup"() -> (w1139:string)
            n545 = Concatenate Strings(w1139, ":Program:Sync") -> (w1141:string)
            n546 = Bundle By Name(cluster=T19 {"Channel Name"="", "New Value"=0.0} ("Update Scan Value Cluster"), "Channel Name"=w1141, "New Value"=1000.0 ("Bundle Element")) -> (w1142:T19)
            n547 = Build Array(w1142) -> (w1144:T19[])
            n548 = call "Update_Current_Value_client.vi"("Update array in"=w1144) -> ()  [unwired: 1 in]
          }
        }
        n549 = Subtract(x=w1130, y=w1129) -> (x-y=w1128:dbl)
        n550 = Greater?(x=w1128, y=300.0) -> (0:w1125:bool)
        n551 = Not(x=w1125) -> (.not. x?=→"Non Starter":bool)
        n552 = Increment(x=w1115) -> (x+1=w1114:T3)
        n553 = Increment(x=w1114) -> (x+1=w1113:T3)
        n554 = Select(t=w1115, s=w1125, f=w1113) -> (s? t:f=w1126:T3)
      }
      frame "Email results to users" {
        n555 = local read "Currently on Row"() -> (w1155:i32)
        n556 = Increment(x=w1155) -> (x+1=w1150:i32)
        n557 = Split 1D Array(array=w1152, index=w1150) -> (first subarray=w1159:T6[], second subarray=w1158:T6[])
        n558 = Array Size(array=w1158) -> (size(s)=w1160:i32)
        n559 = for {
          tunnel: w1159 -> [w1175] mode=indexing
          shift-right: [w1173] -> w1161
          shift-left: string[] [] -> [w1174]
          n560 = Unbundle By Name(w1175) -> ("Row Type Selector"=w1166:T8, "Filename"=w1172:path, "Comments"=w1171:string)
          n561 = Not Equal?(x=Multi_run_mode."Auto Calibrate" ("Row Type Selector"), y=w1166) -> (x != y?=w1168:bool)
          n562 = Empty String/Path?(string/path=w1172) -> (empty?=w1169:bool)
          n563 = Compound Arithmetic op=AND(w1168, invert w1169) -> (w1167:bool)
          n564 = case shown="True" w1167 {
            tunnel: w1174 -> [w1176 w1184]
            tunnel: [w1176 w1183] -> w1173
            tunnel: w1172 -> [_ w1182]
            tunnel: w1171 -> [_ w1180]
            frame False {
            }
            frame True {
              n565 = Path To String(path=w1182) -> (string=w1181:string)
              n566 = Match Pattern(string=w1180, regular expression=" !!Program added comments") -> (after substring=w1177:string)  [unwired: 4 out]
              n567 = Concatenate Strings(w1181, w1177) -> (w1179:string)
              n568 = Build Array (concatenate)(w1184, w1179) -> (w1183:string[])
            }
          }
        }
        n569 = Equal To 0?(x=w1160) -> (x = 0?=w1151:bool)
        n570 = case shown="False" w1151 {
          tunnel: ["Having completed only some of the requested rows." ("Message") ""] -> w1156
          frame False {
          }
          frame True {
          }
        }
        n571 = call "End_of_run_messages.vi"("Message"=w1156, "Subject"="Multi Run Ended", "Attachments"=w1161) -> ()  [unwired: 1 in]
      }
      frame "Save run efficiency" {
        w1198 = FALSE  # append to file? (new file:F)
        w1197 = FALSE  # advisory dialog? (display:T)
        n572 = call "Get_IP_Number.vi"() -> ("Computer Name"=w1186:string)  [unwired: 1 out]
        n573 = Format Into String(format string="Preferences_%s.xls" ("name or relative path"), w1186) -> (resulting string=w1185:string)  [unwired: 2 in, 1 out]
        n574 = call "Setup_Filepath.vi"("Setup File Type"=Setup_Filetype."General", "Filename in"=w1185) -> ("Filename Out"=w1188:path)  [unwired: 1 out]
        n575 = call "Overhead_Factor.vi"("Mode"=Overhead."Read Current Overhead") -> ("Current Overhead Factor"=w1192:dbl)  [unwired: 3 in]
        n576 = Number To Fractional String(number=w1192, precision (6)=i16 4) -> (F-format string=w1190:string)  [unwired: 2 out]
        n577 = call "Read_Characters_From_File.ph.vi"("file path (dialog if empty)"=w1188) -> ("character string"=w1195:string)  [unwired: 1 in, 7 out]
        n578 = call "Replace_data_in_setup_string.vi"("New data string"=w1190, "Input string"=w1195, "Variable name"="Current Overhead Factor") -> ("Appended string"=w1194:string)
        n579 = call "Write_Characters_To_File.vi"("file path (dialog if empty)"=w1188, "advisory dialog? (display:T)"=w1197, "character string"=w1194, "append to file? (new file:F)"=w1198) -> ()  [unwired: 1 in, 4 out]
      }
      frame "Remove Skipped Commands" {
        n580 = for {
          tunnel: w1204 -> [w1212] mode=indexing
          tunnel: [w1211] -> w1203 mode=indexing
          n581 = Unbundle By Name(w1212) -> ("Comments"=w1210:string)
          n582 = Match Pattern(string=w1210, regular expression=" !!Program added comments") -> (before substring=w1209:string)  [unwired: 4 out]
          n583 = Bundle By Name(cluster=w1212, "Comments"=w1209) -> (w1211:T6)
        }
      }
      frame "Show jumped positions" {
        n584 = global read "Trav_pos_global.vi" "Jumped Positions"() -> (w1215:dbl[][])
        n585 = Array Size(array=w1215) -> (size(s)=w1218:i32[])
        n586 = Index Array(array=w1218, index=0) -> (element=w1214:i32)
        n587 = Greater Than 0?(x=w1214) -> (x > 0?=w1216:bool)
        n588 = case shown="True" w1216 {
          tunnel: w1215 -> [_ w1229]
          tunnel: w1214 -> [_ w1228]
          frame False {
            w1222 = TRUE  # Front Panel Window:Is Frontmost
            n589 = Current VI's Path() -> (path=w1223:path)
            n590 = Open VI Reference(vi path=w1223) -> (vi reference=w1224:refnum<vi>, error out=w1225:errorcluster)  [unwired: 1 in, 4 out]
            n591 = property class="VI"(reference=w1224, error in=w1225, "Front Panel Window:Is Frontmost"=w1222) -> (reference out=w1226:refnum<vi>, error out=w1227:errorcluster)
            n592 = Close Reference(reference=w1226, error in (no error)=w1227) -> ()  [unwired: 1 out]
          }
          frame True {
            n593 = stacked-sequence {
              tunnel: w1229 -> [w1230 w1240]
              tunnel: w1228 -> [w1234 _]
              frame #0 {
                n594 = global read "Trav_pos_global.vi" "Default Traverse Setup"() -> (w1231:string)
                n595 = Format Into String(format string="There are %d points which cannot be reached", w1234) -> (resulting string=w1232:string)  [unwired: 2 in, 1 out]
                n596 = call "Display_Trav_Views.vi"("Current Probe Position"=w1230, "Traverse Name"=w1231, "Open Front Panel"=TRUE, "Error Comments"=w1232, "Crash?"=FALSE) -> ()  [unwired: 2 in, 4 out]
              }
              frame #1 {
                n597 = local read "Command filename"() -> (w1244:path)
                n598 = Array To Spreadsheet String(array=w1240, 3:"%.1f" ("format string")) -> (spreadsheet string=w1238:string)  [unwired: 1 out]
                n599 = Strip Path(path=w1244) -> (stripped path=w1243:path)  [unwired: 1 out]
                n600 = Build Path(base path=w1243, name or relative path="Jumped_Positions.xls") -> (appended path=w1241:path)
                n601 = call "Write_File_Simple.vi"("append to file? (new file:F)"=FALSE, "character string"=w1238, "file path"=w1241) -> ()  [unwired: 2 out]
              }
            }
          }
        }
      }
      frame "Save Setup to File" {
        w1261 = FALSE  # Start of Multi Run Prog
        n602 = Array Size(array=w1275) -> (size(s)=w1280:i32)
        n603 = local read "Last Row Run"() -> (w1250:i32)
        n604 = local read "Status"() -> (w1256:T2)
        n605 = local read "Stop after Repeats"() -> (w1259:bool)
        n606 = local read "stop"() -> (w1260:bool)
        n607 = Decrement(x=w1250) -> (x-1=w1251:i32)
        n608 = local read "Command filename"() -> (w1246:path)
        n609 = Increment(x=w1251) -> (x+1=w1263:i32)
        n610 = Equal?(x=w1256, y=Multi_Run_Status."Continue" ("Status")) -> (x = y?=w1255:bool)
        n611 = Compound Arithmetic op=OR(w1259, w1260, w1255) -> (w1258:bool)
        n612 = local read "Non Starter"() -> (w1268:bool)
        n613 = Select(t=w1263, s=w1258, f=w1251) -> (s? t:f=w1262:i32)
        n614 = Less?(x=w1254, y=T9."Run Multi Run Prog") -> (x < y?=w1252:bool)
        n615 = Equal?(x=w1280, y=w1250) -> (x = y?=w1270:bool)
        n616 = Equal To 0?(x=w1263) -> (x = 0?=w1269:bool)
        n617 = Split 1D Array(array=w1275, index=w1262) -> (second subarray=w1278:T6[])  [unwired: 1 out]
        n618 = Compound Arithmetic op=OR(w1270, w1269, w1268, w1252) -> (w1271:bool)
        n619 = call "Current_Filepath.vi"("Filename in"=w1246, "Data Type"="Commands") -> ("Filename Out"=w1245:path)  [unwired: 1 out]
        n620 = local read "Work in Tunnel Coordinates?"() -> (w1249:T1)
        n621 = local read "Jump Bad Positions"() -> (w1248:bool)
        n622 = case shown="False" w1271 {
          tunnel: w1245 -> [w1288 w1322]
          tunnel: [w1287 w1322] -> w1279
          tunnel: w1278 -> [w1285 _]
          tunnel: [w1284 w1323] -> w1277
          tunnel: w1275 -> [w1286 w1323]
          tunnel: w1249 -> [w1283 _]
          tunnel: w1248 -> [w1282 _]
          frame False {
            n623 = stacked-sequence {
              tunnel: w1288 -> [w1290 w1301 _]
              tunnel: [_ w1294 _] -> w1287
              tunnel: w1286 -> [w1293 _ w1306]
              tunnel: w1285 -> [_ _ w1304]
              tunnel: [_ _ w1303] -> w1284
              tunnel: w1283 -> [w1292 _ _]
              tunnel: w1282 -> [w1291 _ _]
              frame #0 {
                n624 = call "Save_Trav_setup.vi"("Work in Tunnel Coordinates?"=w1292, "Trav Table"=w1293, "Jump Bad Positions"=w1291, "Setup filename"=w1290) -> ()  [unwired: 2 out]
                n625 = global write "Trav_pos_global.vi" "Sync to server now"(TRUE) -> ()
              }
              frame #1 {
                n626 = Strip Path(path=w1301) -> (stripped path=w1302:path, name=w1300:string)
                n627 = call "Add_filename_suffix.vi"("Filename"=w1300) -> ("Original Suffix"=w1297:string, "Base name"=w1299:string)  [unwired: 1 in, 2 out]
                n628 = Concatenate Strings(w1299, "_Rem", w1297) -> (w1296:string)
                n629 = Build Path(base path=w1302, name or relative path=w1296) -> (appended path=w1295:path)
                n630 = call "Find_Unique_Filename.vi"("Path In"=w1295) -> ("Unique Path Out"=w1294:path)  [unwired: 1 in, 1 out]
              }
              frame #2 {
                n631 = Index Array(array=w1306, index=0) -> (element=w1309:T6)
                n632 = Initialize Array(w1309, 0 ("dimension size")) -> (w1308:T6[])
                n633 = global read "Extra_Commands_Global.vi" "Minutes Before Repeating Row"() -> (w1307:string)
                n634 = for {
                  shift-right: [w1312] -> w1305
                  shift-left: w1308 -> [w1314]
                  tunnel: w1307 -> [w1316]
                  tunnel: w1306 -> [w1313] mode=indexing
                  n635 = Unbundle By Name(w1313) -> ("Extra Commands"=w1315:string)
                  n636 = call "Extra_Commands.vi"("String to Search"=w1315, "Command"=w1316) -> ("Command Found"=w1317:bool)  [unwired: 1 in, 4 out]
                  n637 = case shown="False" w1317 {
                    tunnel: w1314 -> [w1318 w1321]
                    tunnel: w1313 -> [_ w1320]
                    tunnel: [w1318 w1319] -> w1312
                    frame False {
                    }
                    frame True {
                      n638 = Build Array (concatenate)(w1321, w1320) -> (w1319:T6[])
                    }
                  }
                }
                n639 = Build Array (concatenate)(w1305, w1304) -> (w1303:T6[])
              }
            }
          }
          frame True {
          }
        }
        n640 = Path To String(path=w1245) -> (string=w1267:string)
        n641 = Concatenate Strings("Multi run Prog Ended having the setup filename of :" ("Message"), w1267) -> (w1266:string)
        n642 = call "Save_Trav_setup.vi"("Work in Tunnel Coordinates?"=w1249, "Trav Table"=w1277, "Jump Bad Positions"=w1248, "Setup filename"=w1279) -> ("Trav Table Out"=w1276:T6[])  [unwired: 1 out]
        n643 = call "Log_Current_row_to_Execute.vi"("Simulate/Run"=w1265, "Message"=w1266, "Start of Multi Run Prog"=w1261) -> ()  [unwired: 2 in, 5 out]
        n644 = Select(t=w1276, s=w1271, f=w1275) -> (s? t:f=w1274:T6[])
      }
      frame "End" {
        w1325 = ""
        w1327 = path ""
        w1328 = 0 ("No. of pts.")
        w1330 = nan
        n645 = global write "Trav_pos_global.vi" "Top level setup filename"(w1327) -> ()
        n646 = global read "Trav_pos_global.vi" "Current Row"() -> (w1334:T6)
        n647 = Bundle By Name(cluster=w1334, "Start X"=w1330, "Start Y"=w1330, "Start Z"=w1330, "End X"=w1330, "End Y"=w1330, "End Z"=w1330, "No. of pts."=w1328, "Spacing"=Spacing."Linear", "Filename"=w1327, "Tunnel Speed"=w1330, "Averaging time (min)"=w1330, "Extra Commands"=w1325, "Specific Arguments"=w1325, "Emission Rate (l/min)"=w1330, "Trace Gas Concentration (%)"=w1330, "Density Ratio"=w1325, "Comments"=w1325, "Row No"=w1328, "Row Type Selector"=Multi_run_mode."Blank Row", "Completion time"=w1325, "Meas Setup File"=w1325, "Row Duration (mins)"=w1330, "No. of Valid pts."=w1328) -> (w1333:T6)
        n648 = Current VI's Path() -> (path=w1326:path)
        n649 = global write "Trav_pos_global.vi" "Current Row"(w1333) -> ()
        n650 = global write "Trav_pos_global.vi" "Meas Setup Number"(0 ("Meas Setup Number")) -> ()
        n651 = call "Bring_to_front.vi"("path"=w1326) -> ()
        n652 = global write "Trav_pos_global.vi" "Estimated Completion time"("") -> ()
        n653 = Build Array(u32 0) -> (w1335:u32[])
        n654 = property on="Table" class="Arr (strict)"("Index Values"=w1335) -> ()  [unwired: 2 in, 2 out]
      }
    }
    n655 = case shown="True" w8 {
      tunnel: w4 -> [_ w15]
      frame False {
      }
      frame True {
        n656 = local write "Table"(w15) -> ()
      }
    }
    "Multi Run Case" <- w10
  }
